vi "UHR-Fleezers Control (fpga) - 10.9.vi"() -> ()   [LabVIEW 2014]
doc: "UHR-Fleezers Instrument Control Code (fpga)"
uses:
  <vilib>/eio/EIONode/EIONode.xnode
  <vilib>/eio/EIOMethodNode/EIOMethodNode.xnode
  <vilib>/rvi/DataTransferAndStorage/Container/XNode/niFpgaContainer.xnode
  <vilib>/Platform/TimedLoop/XDataNode/XDataNode.xnode
  <vilib>/Platform/TimedLoop/XDataNode/nitl_modes.ctl
  <vilib>/Platform/TimedLoop/XDataNode/XDNodeRunTimeDep.lvlib
  <vilib>/Platform/TimedLoop/XDataNode/wakeup.ctl
  <vilib>/Platform/TimedLoop/XDataNode/timing_clust.ctl
  <vilib>/addons/control/pid/fpga.llb/XNode/niFpgaPID.xnode
  <vilib>/rvi/eio/common/nirviEmuTemplateMethod_errors.vi
  <vilib>/rvi/interface/RandomDataEmulation/nirviRandomDataFpgaReadWriteTemplate.vi
panel:
  in  "Connector0/AO6":i16
  in  "Tab Control":T1(tab)=enum."Force FB"
  in  "Trap Pos to FIFO":bool
  in  "AI1 Sets to FIFO":T2={"Set 1"=TRUE, "Set 2"=TRUE, "Set 3"=FALSE}
  in  "N of AI1 Int Acq Sets":i16=2 min=1 max=3 step=1
  out "AI Late Counter":u8
  in  "ai count":u16=400
  in  "+ phase":bool
  in  "Phase count adjustment":i16
  out "Relative phase":i16
  in  "AI to FIFO":bool
  out "BD1 Frequency Out 1":u64
  out "BD1 Frequency Out 2":u64
  out "Trap Pos FIFO Timeout":u16
  out "Trap AI FIFO Timeout":u16
  in  "Trap FIFO Set Timeout":i32
  in  "Tab Control 2":T3(tab)
  out "Wiggling 2":bool
  in  "Abort wiggle 2":bool
  in  "Wiggle amp 2":u64
  in  "Wiggle freq 2 (Hz)":fxp<+/-,16,16>
  in  "Wiggle trap 2":bool
  out "Wiggling 1":bool
  in  "Abort wiggle 1":bool
  in  "Wiggle trap 1":bool
  in  "Wiggle amp 1":u64
  in  "Wiggle freq 1 (Hz)":fxp<+/-,16,16>
  in  "Swap F1 and F2":bool
  in  "Freq or Amp switch first":bool=TRUE
  in  "Cont. Scan":bool
  in  "Abort scan":bool
  in  "Cycles per step":u64
  in  "Scan BD":bool
  in  "Number of scans":u16
  in  "Scan steps":u64
  in  "Scan freq.  increment":i64
  out "Scanning":bool
  in  "Start scan":bool
  in  "OSK Bd 1":bool
  in  "Reset Bd 1":bool
  in  "RD":bool
  in  "PMODE":bool
  in  "OSK Bd 2":bool
  in  "Reset Bd 2":bool
  in  "Direct RF Box \nCommunication":bool
  in  "Data BD 2":u8 format="%08b"
  in  "Data BD 1":u8 format="%08b"
  in  "Address":u8 format="%02x"
  in  "Update Data":bool
  in  "FPGA Controls\n RF Box":bool
  in  "Number Interlace Cycles":u8=2 min=1 max=3
  in  "Interlace Off Parameters":u8=1 min=1 max=3
  in  "Interlace ON/OFF":bool
  out "DIO Relative phase":i16
  in  "Phase count adjustment (DIO)":i16
  in  "+ phase (DIO)":bool
  out "DIO Late Counter":u8
  in  "DIO count 1 (ticks)":u16=400
  in  "DIO count 2 (ticks)":u16=400
  in  "DIO count 3 (ticks)":u16=400
  out "AI2 Y Sum Set 2":i16
  out "AI2 Y Sum Set 1":i16
  in  "FB Gains Set 1":T4={"proportional gain (Kc)"=10, "integral gain (Kc*Ts/Ti)"=5, "derivative gain (Kc*Td/Ts)"=0}
  in  "FB Setpoint Set 1":i16 min=0 step=1
  in  "FB Reset Set 1":bool
  in  "FB On/Off Set 1":bool
  in  "FB Reset Set 2":bool
  in  "FB On/Off Set 2":bool
  in  "FB Setpoint Set 2":i16 min=0 step=1
  in  "FB Gains Set 2":T4={"proportional gain (Kc)"=10, "integral gain (Kc*Ts/Ti)"=5, "derivative gain (Kc*Td/Ts)"=0}
  in  "FB output range 2":cluster{"output high":i16, "output low":i16}={"output high"=3000, "output low"=0}
  in  "FB output range 1":cluster{"output high":i16, "output low":i16}={"output high"=3000, "output low"=0}
  out "Scan I":u64
  in  "Amp switch delay":u16=5
  in  "Freq switch delay":u16
  in  "BD 2 Amplitude 1":u16
  in  "BD 1 Amplitude 1":u16
  in  "BD 2 Frequency 1":u64
  in  "BD 1 Frequency 1":u64
  in  "BD 2 Amplitude 2":u16
  in  "BD 1 Amplitude 2":u16
  in  "BD 2 Frequency 2":u64
  in  "BD 1 Frequency 2":u64
  in  "BD 2 Amplitude 3":u16
  in  "BD 1 Amplitude 3":u16
  in  "BD 2 Frequency 3":u64
  in  "BD 1 Frequency 3":u64
  in  "Negate Diff?":bool
  in  "Diff FB Measurement?":bool
  in  "FB Trig Integrate":u32=1
  out "TTrig?":bool
  in  "TTrig Negate Pos":bool=TRUE
  out "Trap Pos FB Int Signal":fxp<+/-,24,9> format="%.18g"
  out "Trap Pos FB Int-Norm Signal":fxp<+/-,16,1> format="%.16g"
  in  "FPGA TTrig Thresh":i64
  in  "FPGA Trap Trig":bool
  out "Trap Pos FB Action":i64
  in  "Trap Pos. FB Offset Factor":i64
  in  "Trap Pos. FB Mult Factor":i64=2
  in  "Trap Pos. FB Range":T5={"output high"=0.999969482421875, "output low"=-1.0}
  in  "Trap Pos. FB Gains":T6={"proportional gain (Kc)"=0.0, "integral gain (Kc*Ts/Ti)"=10.0, "derivative gain (Kc*Td/Ts)"=0.0} {"proportional gain (Kc)" format="%.11g"; "integral gain (Kc*Ts/Ti)" format="%.11g"; "derivative gain (Kc*Td/Ts)" format="%.11g"}
  in  "Trap Pos. FB Reset":bool
  in  "Trap Pos FB Monitor T1 or T2":bool
  in  "AI1 X Scale":u16
  in  "Trap Pos FB Int Count":u16=100
  in  "Trap Pos FB Negate Action":bool
  out "AI1 X Set 2":fxp<+/-,16,1>
  out "AI1 X Set 1":fxp<+/-,16,1>
  in  "Trap Pos. FB SP":fxp<+/-,16,1>
  in  "Force feedback":bool
  out "TTrig Sig":i64
  out "TTrig Fin Thresh":i64
  out "Numeric":i32
  out "AO2 2":i16
  out "AO1 2":i16
  in  "1D or 2D Scan?":bool
  in  "Abort scan (MCL)":bool
  in  "MCL Scan Axis":bool
  in  "Cont. Scan (MCL)":bool
  out "Scan I (MCL)":u64
  in  "Number of scans (MCL)":u16
  out "Scanning MCL":bool
  in  "Scan steps (MCL)":u64
  in  "Cycles per step (MCL)":u64
  in  "Scan freq.  increment (MCL)":i16
  in  "Start scan (MCL)":bool
  in  "AO2":i16
  in  "AO1":i16
  out "MCL Late Counter":u8
  in  "MCL count":u32=800
  out "MCL Relative Phase":i16
  in  "Phase count adjustment (MCL)":i16
  in  "+ phase (MCL)":bool
  in  "APD Gate Operating Mode":u8 max=2 step=1
  in  "Invert APD Gate":bool
  in  "APD Gate OFF Count":u16=100
  in  "APD Gate ON Count":u16=300
  out "APD 1 Gate Late Counter":u8
  out "APD 1 Gate Relative Phase":i16
  in  "Phase count adjustment (APD 1 Gate)":i16
  in  "+ phase (APD 1 Gate)":bool
  out "APD 2 Counts 0":u32
  out "APD 2 Counts 1":u32
  out "APD 1 Counts 0":u32
  out "APD 1 Counts 1":u32
  out "APD 1 out state":bool
  in  "APD 2 AO scale factor":i16=1
  in  "APD 1 AO scale factor":i16=1
  in  "APD to FIFO":bool
  in  "APD Acq Rate Count":u32=20000000
  out "APD Acq Late Counter":u8
  out "APD Acq Relative Phase":i16
  in  "Phase Count Adjustment (APD Acq)":i16
  in  "+ phase (APD Acq)":bool
  in  "Phase count adjustment (APD 2 Gate)":i16
  out "APD 2 Gate Late Counter":u8
  out "APD 2 Gate Relative Phase":i16
  in  "+ phase (APD 2 Gate)":bool
  out "APD 2 out state":bool
  out "APD 1 Int Gate":bool
  out "APD 2 Int Gate":bool
  in  "Green Filter Flipper":bool
  out "Green FB Signals":T7
  in  "Green FB Count":u16=1200
  out "Green Late Counter":u8
  out "Green FB Relative Phase":i16
  in  "Phase count adjustment (Green FB)":i16=10
  in  "+ phase (Green FB)":bool
  out "Green FB Sum":i16
  in  "Green int current ON count adj":u16=150
  in  "Current Out":u16=30000
  in  "Green FB On/Off":bool
  in  "Green FB Setpoint":i16=250 min=0 step=1
  in  "Green FB Gains":T4={"proportional gain (Kc)"=10, "integral gain (Kc*Ts/Ti)"=5, "derivative gain (Kc*Td/Ts)"=0}
  in  "Green FB Reset":bool
  in  "Operating Mode 2":u8=2 max=2 step=1
  in  "Invert GI 2":bool
  in  "Green interlace OFF count 2":u16=900
  in  "Green interlace ON count 2":u16=300
  out "GI Late Counter 2":u8
  out "GI Relative phase 2":i16
  in  "Phase count adjustment (GI) 2":i16=20
  in  "+ phase (GI) 2":bool
  in  "Green interlace OFF count":u16=100
  out "GI Relative phase":i16
  in  "Phase count adjustment (GI)":i16
  in  "+ phase (GI)":bool
  in  "Green interlace ON count":u16=300
  out "GI Late Counter":u8
  in  "Invert GI":bool
  in  "Operating Mode":u8 max=2 step=1
  in  "Red FB Reset":bool
  in  "Red FB Setpoint":i16
  in  "Red FB On/Off":bool
  in  "Invert RI 2":bool
  in  "Invert RI":bool
  in  "Phase count adjustment (RI)":i16
  in  "+ phase (RI)":bool
  in  "RI OFF count":u16
  in  "RI ON count":u16
  in  "RI Current Out":u16
  in  "RI operating mode 2":u8
  in  "Red operating mode":u8
  out "RI late counter":u8
  out "RI relative phase":i16
  out "Red FB Sum":i16
  in  "Red FB Gains":T4={"proportional gain (Kc)"=1, "integral gain (Kc*Ts/Ti)"=0, "derivative gain (Kc*Td/Ts)"=0}
  in  "Chassis2/Mod4/AO1":u16
  # "Only one of these can be on\nat a time:"
  # "Raster Scan AOD"
  # "1 (X)"
  # "2 (Y)"
  # "IR Intensity Feedback (RF BD 1)"
  # "FB Triggering Excitation Laser"
  # "AO1 (Y)"
  # "2D"
  # "1D"
  # "AO2 (X)"
  # "APD AO for aligning"
  # "Detection Loop"
  # "Green fluorescent laser digital gate interlacing loop"
  # "0 Forced ON\n1 Forced OFF\n2 Interlacing"
  # "Red fluorescent laser digital gate interlacing loop"
  # "0 Forced ON\n1 Forced OFF\n2 Interlacing"
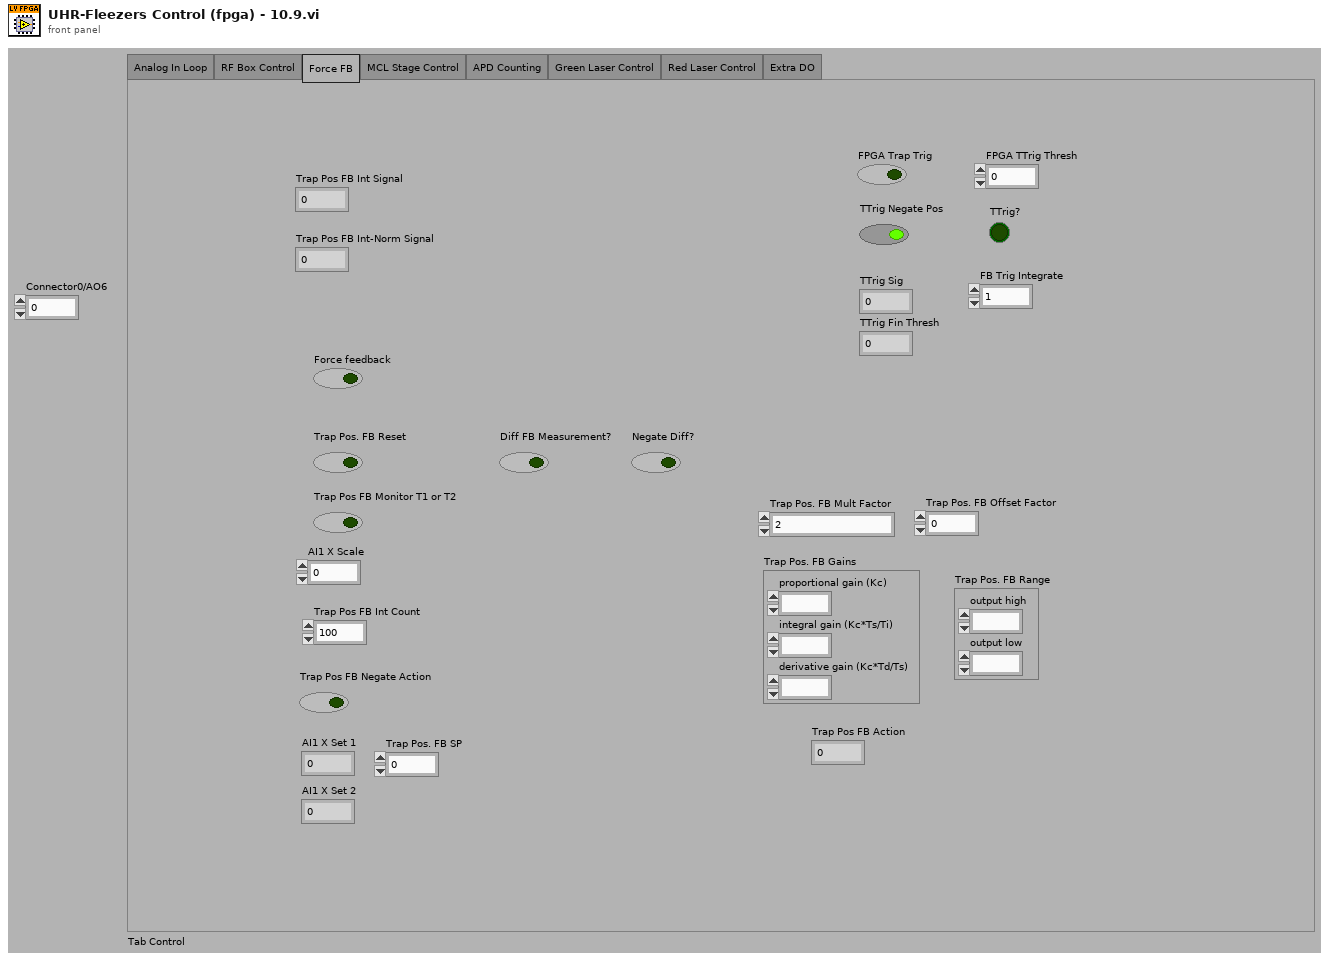
[diagram p1: front panel]
types:
  T1 = enum32{"Analog In Loop", "RF Box Control", "Force FB", "MCL Stage Control", "APD Counting", "Green Laser Control", "Red Laser Control", "Extra DO"}
  T2 = cluster{"Set 1":bool, "Set 2":bool, "Set 3":bool}
  T3 = enum32{"Controls", "Interlacing Frequency and Amplitude Values"}
  T4 = cluster{"proportional gain (Kc)":i16, "integral gain (Kc*Ts/Ti)":i16, "derivative gain (Kc*Td/Ts)":i16}
  T5 = cluster{"output high":fxp<+/-,16,1>, "output low":fxp<+/-,16,1>}
  T6 = cluster{"proportional gain (Kc)":fxp<+/-,16,8>, "integral gain (Kc*Ts/Ti)":fxp<+/-,16,8>, "derivative gain (Kc*Td/Ts)":fxp<+/-,16,8>}
  T7 = cluster{"Green FB Ch 0":i16, "Green FB Ch 1":i16, "Green FB Ch 2":i16}
  T8 = typedef "XDNodeRunTimeDep.lvlib/timing_clust.ctl" = cluster{"Expected End [f-1]":u64, "Actual End [f-1]":u64, "Finished Late? [f-1]":bool, "Expected End [i-1]":u64, "Actual End [i-1]":u64, "Finished Late? [i-1]":bool, "Expected Start [i]":u64, "Actual Start [i]":u64, "Expected Start [f]":u64, "Actual Start [f]":u64, "Source Name":string, "Structure Name":string, "Period":i64, "Deadline":i64, "Offset":i64, "Start":i64, "Priority":i32, "Timeout":i32, "Mode":T9, "Wakeup Reason":T10, "Error":errorcluster, "Source Type":string, "Secondary Source Type":string, "Global End Time":u64, "Global Start Time":u64, "Frame Duration":u64, "Iteration Duration":u64, "Assigned CPU":i32, "I/O Scan Engine Mode":u32}
  T9 = typedef "XDNodeRunTimeDep.lvlib/nitl_modes.ctl" = enum32{"No Change", "Process missed periods, maintain original phase", "Discard missed periods, maintain original phase", "Process missed periods, ignore original phase", "Discard missed periods, ignore original phase"}
  T10 = typedef "XDNodeRunTimeDep.lvlib/wakeup.ctl" = enum32{"Normal", "Aborted", "Asynchronous wakeup", "Timing source error", "Timed loop error", "Timeout"}
  T11 = cluster{"Chassis2/Mod1/AI0":void, "Chassis2/Mod1/AI1":void, "Chassis2/Mod1/AI2":void}
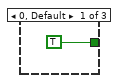
[diagram p2: hidden frame]
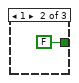
[diagram p3: hidden frame]
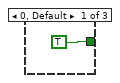
[diagram p4: hidden frame]
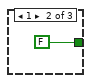
[diagram p5: hidden frame]
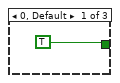
[diagram p7: hidden frame]
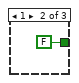
[diagram p8: hidden frame]
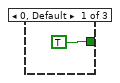
[diagram p10: hidden frame]
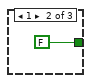
[diagram p11: hidden frame]
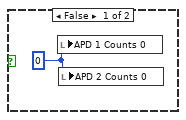
[diagram p12: hidden frame]
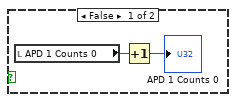
[diagram p15: hidden frame]
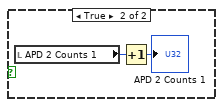
[diagram p17: hidden frame]
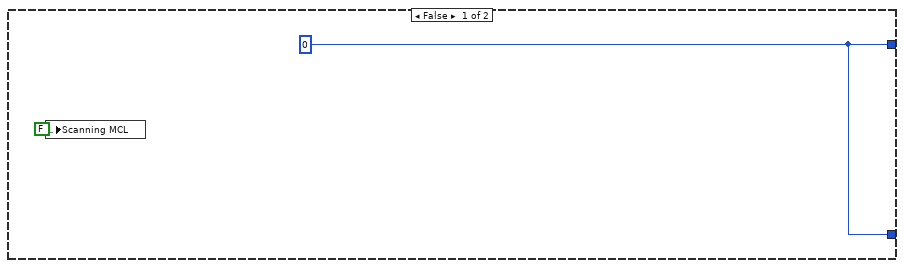
[diagram p18: hidden frame]
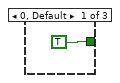
[diagram p19: hidden frame]
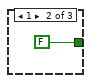
[diagram p20: hidden frame]
diagram:
  w1 = u16 0
  w4 = FALSE
  w2 = FALSE
  # "633 nm red excitation laser interlacing (DO to IA 633 nm AOM ME amp)."
  # "The APD Int Gate is here so the FPGA will do the integration only when the APD gate is \"ON\" (though we will leave the APD continuously ON now). This was added because the actual APD gating (via the hardware) was giving false signals. -KW"
  # "timing array current index"
  # "timing array"
  # "timing counter (phase adjusted here)"
  # "late counter"
  n1 = flat-sequence "FPGA initialization to do before running any of the loops" {
    tunnel: [u16 0 ("DIO count 3 (ticks)")] -> w3
    tunnel: [w10] -> _
    frame #0 {
      # "Start up expansion chassis early\nto avoid delays later"
      # "This pin controls udclk on the RF boards.\nWhen initially configuring the boards, this pin needs to be\nconfigured as a high impedance input.  Later it will be switched\nto an output."
      # "Initial setting of DIO data and \naddress to low (before reset).  \nThis needs to happen before the other\ncontrol method loops execute."
      n2 = xnode "FPGA I/O Node"("Chassis2/Mod4/AO0"=u16 0) -> ("Chassis2/Mod1/AI0"=w10)  [unwired: 2 in, 2 out]
      n3 = xnode "FPGA I/O Method Node"("Enable"=FALSE) -> ()  [unwired: 1 in, 1 out]
      n4 = xnode "FPGA I/O Node"("Connector1/DIO0"=FALSE, "Connector1/DIO1"=FALSE, "Connector1/DIO2"=FALSE, "Connector1/DIO3"=FALSE, "Connector1/DIO4"=FALSE, "Connector1/DIO5"=FALSE, "Connector1/DIO6"=FALSE, "Connector1/DIO7"=FALSE, "Connector1/DIO8"=FALSE, "Connector1/DIO9"=FALSE, "Connector1/DIO10"=FALSE, "Connector1/DIO11"=FALSE, "Connector1/DIO12"=FALSE, "Connector1/DIO13"=FALSE, "Connector1/DIO15"=FALSE, "Connector1/DIO20"=FALSE, "Connector1/DIO21"=FALSE, "Connector1/DIO22"=FALSE, "Connector1/DIO23"=FALSE, "Connector1/DIO24"=FALSE, "Connector1/DIO25"=FALSE, "Connector1/DIO26"=FALSE, "Connector1/DIO27"=FALSE, "Connector1/DIO14"=FALSE) -> ()  [unwired: 24 in, 24 out]
    }
  }
  n5 = local read "AO1"() -> (w8:i16)
  n6 = local read "AO2"() -> (w7:i16)
  n7 = node-c288() -> (w6:T8)  [unwired: 1 in]
  n8 = while "APD 1 Counter" {
    tunnel: w3 -> [_]
    stop <- FALSE stop-if-true
    n9 = flat-sequence {
      frame #0 {
        n10 = xnode "FPGA I/O Method Node"("FPGA I/O In"=refnum<k21> "Connector0/DIO0" ("APD 1 DO"), "Timeout"=-1) -> ()  [unwired: 2 out]
      }
      frame #1 {
        n11 = local read "APD 1 Int Gate"() -> (w41:bool)
        n12 = case shown="True" w41 {
          frame False {
          }
          frame True {
            n13 = local read "APD 1 out state"() -> (w42:bool)
            n14 = case shown="True" w42 {
              frame False {
                n15 = local read "APD 1 Counts 0"() -> (w44:u32)
                n16 = Increment(x=w44) -> (x+1=→"APD 1 Counts 0":u32)
              }
              frame True {
                n17 = local read "APD 1 Counts 1"() -> (w46:u32)
                n18 = Increment(x=w46) -> (x+1=→"APD 1 Counts 1":u32)
              }
            }
          }
        }
      }
    }
  }
  n19 = while "APD 2 Counter" {
    tunnel: w3 -> [_]
    stop <- FALSE stop-if-true
    n20 = flat-sequence {
      frame #0 {
        n21 = xnode "FPGA I/O Method Node"("FPGA I/O In"=refnum<k21> "Connector0/DIO1" ("APD 2 DO"), "Timeout"=-1) -> ()  [unwired: 2 out]
      }
      frame #1 {
        n22 = local read "APD 2 Int Gate"() -> (w50:bool)
        n23 = case shown="True" w50 {
          frame False {
          }
          frame True {
            n24 = local read "APD 2 out state"() -> (w51:bool)
            n25 = case shown="False" w51 {
              frame False {
                n26 = local read "APD 2 Counts 0"() -> (w53:u32)
                n27 = Increment(x=w53) -> (x+1=→"APD 2 Counts 0":u32)
              }
              frame True {
                n28 = local read "APD 2 Counts 1"() -> (w55:u32)
                n29 = Increment(x=w55) -> (x+1=→"APD 2 Counts 1":u32)
              }
            }
          }
        }
      }
    }
  }
  n30 = while "APD 2 Gating" {
    shift-right: [w59] -> _
    shift-left: w3 -> [w64]
    shift-right: [w58] -> _
    shift-left: w4 -> [w56]
    stop <- FALSE stop-if-true
    n31 = flat-sequence {
      tunnel: w64 -> [w67]
      tunnel: [w68] -> w62
      tunnel: [w67] -> w60
      tunnel: [w66] -> w57
      tunnel: w56 -> [w66]
      tunnel: [w71] -> w63
      tunnel: w62 -> [w71]
      tunnel: [w70] -> w61
      tunnel: w60 -> [w70]
      tunnel: w57 -> [w69]
      tunnel: [w89] -> w59
      tunnel: w63 -> [w100]
      tunnel: w61 -> [w98]
      tunnel: [w93] -> w58
      frame #0 {
        n32 = call "Loop Timer8"("Count(Ticks)"=w67) -> ("Tick Count(Ticks)"=w68:u16)
      }
      frame #1 {
        # "(need 4 channels/APD)"
        n33 = xnode "FPGA I/O Node"("Connector0/DIO8"=w69, "Connector0/DIO9"=w69, "Connector0/DIO10"=w69, "Connector0/DIO11"=w69) -> ()  [unwired: 4 in, 4 out]
        "APD 2 Int Gate" <- w69
      }
      frame #2 {
        n34 = local read "APD Gate ON Count"() -> (w82:u16)
        n35 = local read "APD Gate OFF Count"() -> (w81:u16)
        n36 = feedback #1(TRUE) -> (w95:bool)
        n37 = feedback-in #2(w100) -> ()
        n38 = feedback #2(w100) -> (w83:u16)
        n39 = Not(x=w95) -> (.not. x?=w92:bool)
        n40 = feedback-in #1(w92) -> ()
        n41 = Subtract(x=w100, y=w83) -> (x-y=w99:u16)
        n42 = Select(t=w82, s=w92, f=w81) -> (s? t:f=w97:u16)
        n43 = Subtract(x=w99, y=w98) -> (x-y=w74:u16)
        n44 = Subtract(x=w97, y=w74) -> (x-y=w88:u16)
        n45 = Number To Boolean Array(number=w74) -> (Boolean array=w73:bool[])
        n46 = Or Array Elements(Boolean array=w73) -> (logical OR=w72:bool)
        n47 = Boolean To (0,1)(Boolean="+ phase (APD 2 Gate)") -> (0, 1=w86:i16)
        n48 = Multiply(x=w86, y="Phase count adjustment (APD 2 Gate)") -> (x*y=w84:i16)
        n49 = Boolean To (0,1)(Boolean=w72) -> (0, 1=w79:i16)
        n50 = Add(x=w88, y=w84) -> (x+y=w89:u16)
        n51 = To Unsigned Byte Integer(number=w79) -> (unsigned 8bit integer=w76:u8)
        n52 = feedback #3(i16 0) -> (w91:i16)
        n53 = Subtract(x=w91, y=w84) -> (x-y=w90:i16)
        "APD 2 Gate Relative Phase" <- w90
        n54 = feedback-in #3(w90) -> ()
        n55 = feedback #4(u8 0) -> (w77:u8)
        n56 = Add(x=w76, y=w77) -> (x+y=w75:u8)
        "APD 2 Gate Late Counter" <- w75
        n57 = feedback-in #4(w75) -> ()
        n58 = local read "APD Gate Operating Mode"() -> (w80:u8)
        n59 = case shown="2" w80 {
          tunnel: [TRUE FALSE w106] -> w93
          tunnel: w95 -> [_ _ w104]
          frame 0, Default {
          }
          frame 1 {
          }
          frame 2 {
            n60 = local read "Invert APD Gate"() -> (w103:bool)
            n61 = Not(x=w104) -> (.not. x?=w105:bool)
            n62 = Select(t=w105, s=w103, f=w104) -> (s? t:f=w106:bool)
          }
        }
      }
    }
  }
  n63 = while "APD 1 Gating" {
    shift-right: [w110] -> _
    shift-left: w3 -> [w115]
    shift-right: [w109] -> _
    shift-left: w4 -> [w107]
    stop <- FALSE stop-if-true
    n64 = flat-sequence {
      tunnel: w115 -> [w118]
      tunnel: [w119] -> w113
      tunnel: [w118] -> w111
      tunnel: [w117] -> w108
      tunnel: w107 -> [w117]
      tunnel: [w122] -> w114
      tunnel: w113 -> [w122]
      tunnel: [w121] -> w112
      tunnel: w111 -> [w121]
      tunnel: w108 -> [w120]
      tunnel: [w136] -> w110
      tunnel: w114 -> [w151]
      tunnel: w112 -> [w148]
      tunnel: [w140] -> w109
      frame #0 {
        n65 = call "Loop Timer7"("Count(Ticks)"=w118) -> ("Tick Count(Ticks)"=w119:u16)
      }
      frame #1 {
        # "(need 4 channels/APD)"
        n66 = xnode "FPGA I/O Node"("Connector0/DIO4"=w120, "Connector0/DIO5"=w120, "Connector0/DIO6"=w120, "Connector0/DIO7"=w120) -> ()  [unwired: 4 in, 4 out]
        "APD 1 Int Gate" <- w120
      }
      frame #2 {
        n67 = feedback #5(TRUE) -> (w143:bool)
        n68 = feedback-in #6(w151) -> ()
        n69 = feedback #6(w151) -> (w150:u16)
        n70 = Not(x=w143) -> (.not. x?=w139:bool)
        n71 = feedback-in #5(w139) -> ()
        n72 = Subtract(x=w151, y=w150) -> (x-y=w149:u16)
        n73 = Select(t="APD Gate ON Count", s=w139, f="APD Gate OFF Count") -> (s? t:f=w145:u16)
        n74 = Subtract(x=w149, y=w148) -> (x-y=w124:u16)
        n75 = Subtract(x=w145, y=w124) -> (x-y=w135:u16)
        n76 = Number To Boolean Array(number=w124) -> (Boolean array=w125:bool[])
        n77 = Or Array Elements(Boolean array=w125) -> (logical OR=w123:bool)
        n78 = Boolean To (0,1)(Boolean="+ phase (APD 1 Gate)") -> (0, 1=w133:i16)
        n79 = Boolean To (0,1)(Boolean=w123) -> (0, 1=w130:i16)
        n80 = Multiply(x=w133, y="Phase count adjustment (APD 1 Gate)") -> (x*y=w131:i16)
        n81 = To Unsigned Byte Integer(number=w130) -> (unsigned 8bit integer=w127:u8)
        n82 = Add(x=w135, y=w131) -> (x+y=w136:u16)
        n83 = feedback #7(i16 0) -> (w138:i16)
        n84 = Subtract(x=w138, y=w131) -> (x-y=w137:i16)
        "APD 1 Gate Relative Phase" <- w137
        n85 = feedback-in #7(w137) -> ()
        n86 = feedback #8(u8 0) -> (w128:u8)
        n87 = Add(x=w127, y=w128) -> (x+y=w126:u8)
        "APD 1 Gate Late Counter" <- w126
        n88 = feedback-in #8(w126) -> ()
        n89 = case shown="2" "APD Gate Operating Mode" {
          tunnel: [TRUE FALSE w157] -> w140
          tunnel: w143 -> [_ _ w154]
          frame 0, Default {
          }
          frame 1 {
          }
          frame 2 {
            n90 = Not(x=w154) -> (.not. x?=w156:bool)
            n91 = Select(t=w156, s="Invert APD Gate", f=w154) -> (s? t:f=w157:bool)
          }
        }
      }
    }
  }
  n92 = timed-loop "RF box board DIO control: control bits" {
    timing: w6 -> [_]
    timing-out: [_] -> w5
    tunnel: [w158] -> _
    tunnel: w3 -> [w158]
    stop <- FALSE stop-if-true
    n93 = xnode "FPGA I/O Node"("Connector1/DIO16"="RD", "Connector1/DIO17"="PMODE", "Connector1/DIO18"="OSK Bd 1", "Connector1/DIO19"="Reset Bd 1", "Connector1/DIO28"="OSK Bd 2", "Connector1/DIO29"="Reset Bd 2") -> ()  [unwired: 6 in, 6 out]
  }
  n94 = while "532 nm green excitation laser interlacing (DO to IA 532 nm AOM ME amp)." {
    shift-right: [w171] -> _
    shift-left: w3 -> [w176]
    shift-right: [w170] -> _
    shift-left: w2 -> [w168]
    stop <- FALSE stop-if-true
    n95 = flat-sequence {
      tunnel: w176 -> [w179]
      tunnel: [w180] -> w174
      tunnel: [w179] -> w172
      tunnel: [w178] -> w169
      tunnel: w168 -> [w178]
      tunnel: [w183] -> w175
      tunnel: w174 -> [w183]
      tunnel: [w182] -> w173
      tunnel: w172 -> [w182]
      tunnel: w169 -> [w181]
      tunnel: [w192] -> w171
      tunnel: w175 -> [w212]
      tunnel: w173 -> [w209]
      tunnel: [w201] -> w170
      frame #0 {
        n96 = call "Loop Timer4"("Count(Ticks)"=w179) -> ("Tick Count(Ticks)"=w180:u16)
      }
      frame #1 {
        n97 = xnode "FPGA I/O Node"("Connector1/DIO37"=w181, "Connector1/DIO38"=w181, "Connector1/DIO39"=w181) -> ()  [unwired: 3 in, 3 out]
      }
      frame #2 {
        n98 = feedback-in #9(w212) -> ()
        n99 = feedback #9(w212) -> (w211:u16)
        n100 = Subtract(x=w212, y=w211) -> (x-y=w210:u16)
        n101 = Subtract(x=w210, y=w209) -> (x-y=w185:u16)
        n102 = Number To Boolean Array(number=w185) -> (Boolean array=w186:bool[])
        n103 = Or Array Elements(Boolean array=w186) -> (logical OR=w184:bool)
        n104 = Boolean To (0,1)(Boolean="+ phase (GI)") -> (0, 1=w197:i16)
        n105 = Multiply(x=w197, y="Phase count adjustment (GI)") -> (x*y=w194:i16)
        n106 = Boolean To (0,1)(Boolean=w184) -> (0, 1=w191:i16)
        n107 = To Unsigned Byte Integer(number=w191) -> (unsigned 8bit integer=w188:u8)
        n108 = feedback #10(i16 0) -> (w195:i16)
        n109 = feedback #11(u8 0) -> (w189:u8)
        n110 = Add(x=w188, y=w189) -> (x+y=w187:u8)
        "GI Late Counter" <- w187
        n111 = feedback-in #11(w187) -> ()
        n112 = Subtract(x=w195, y=w194) -> (x-y=w193:i16)
        "GI Relative phase" <- w193
        n113 = feedback-in #10(w193) -> ()
        n114 = feedback #12(TRUE) -> (w204:bool)
        n115 = case shown="2" "Operating Mode" {
          tunnel: [TRUE FALSE w218] -> w201
          tunnel: w204 -> [_ _ w215]
          frame 0, Default {
          }
          frame 1 {
          }
          frame 2 {
            n116 = Not(x=w215) -> (.not. x?=w217:bool)
            n117 = Select(t=w217, s="Invert GI", f=w215) -> (s? t:f=w218:bool)
          }
        }
        n118 = Not(x=w204) -> (.not. x?=w200:bool)
        n119 = Select(t="Green interlace ON count", s=w200, f="Green interlace OFF count") -> (s? t:f=w206:u16)
        n120 = Subtract(x=w206, y=w185) -> (x-y=w198:u16)
        n121 = Add(x=w198, y=w194) -> (x+y=w192:u16)
        n122 = feedback-in #12(w200) -> ()
      }
    }
  }
  n123 = while "Green and red excitation laser interlacing (Current AO to IA 532 nm AOM ME amp)." {
    shift-right: [w227] -> _
    shift-left: w3 -> [w230]
    shift-right: [w224] -> _
    shift-left: w1 -> [w222]
    shift-right: [w219] -> _
    shift-left: w1 -> [w221]
    stop <- FALSE stop-if-true
    n124 = flat-sequence {
      tunnel: w230 -> [w234]
      tunnel: [w235] -> w229
      tunnel: [w234] -> w228
      tunnel: [w233] -> w223
      tunnel: w222 -> [w233]
      tunnel: w221 -> [w232]
      tunnel: [w232] -> w220
      tunnel: [w239] -> w226
      tunnel: w229 -> [w239]
      tunnel: [w238] -> w225
      tunnel: w228 -> [w238]
      tunnel: w223 -> [w237]
      tunnel: w220 -> [w236]
      tunnel: [w259] -> w227
      tunnel: [w276] -> w224
      tunnel: w226 -> [w245]
      tunnel: w225 -> [w285]
      tunnel: [w247] -> w219
      frame #0 {
        n125 = call "Loop Timer10"("Count(Ticks)"=w234) -> ("Tick Count(Ticks)"=w235:u16)
      }
      frame #1 {
        n126 = xnode "FPGA I/O Node"("Chassis2/Mod4/AO0"=w237, "Chassis2/Mod4/AO1"=w236) -> ()  [unwired: 2 in, 2 out]
      }
      frame #2 {
        # "Design note (Comstock lab):\n\nThese two laser controls are in the same loop\nbecause the expansion current AI cannot separately\ntime the outputs fast enough for us.  Apparently\nit is because of communication time between the\nexpansion card and the fpga.\n\nSo the two analog control signals have the same timing\nand profile, but independent amplitudes to independently\ncontrol the intensity and feedback for each laser."
        n127 = feedback #13(TRUE) -> (w246:bool)
        n128 = Subtract(x="Green interlace OFF count 2", y="Green int current ON count adj") -> (x-y=w268:u16)
        n129 = Not(x=w246) -> (.not. x?=w278:bool)
        n130 = feedback-in #13(w278) -> ()
        n131 = feedback-in #14(w245) -> ()
        n132 = feedback #14(w245) -> (w287:u16)
        n133 = Add(x="Green int current ON count adj", y="Green interlace ON count 2") -> (x+y=w269:u16)
        n134 = Subtract(x=w245, y=w287) -> (x-y=w286:u16)
        n135 = Select(t=w269, s=w278, f=w268) -> (s? t:f=w282:u16)
        n136 = Subtract(x=w286, y=w285) -> (x-y=w252:u16)
        n137 = case shown="2" "RI operating mode 2" {
          tunnel: [TRUE FALSE w301] -> w242
          tunnel: w246 -> [_ _ w303]
          frame 0, Default {
          }
          frame 1 {
          }
          frame 2 {
            n138 = Not(x=w303) -> (.not. x?=w302:bool)
            n139 = Select(t=w302, s="Invert RI 2", f=w303) -> (s? t:f=w301:bool)
          }
        }
        n140 = case shown="2" "Operating Mode 2" {
          tunnel: [TRUE FALSE w321] -> w270
          tunnel: w246 -> [_ _ w318]
          frame 0, Default {
          }
          frame 1 {
          }
          frame 2 {
            n141 = Not(x=w318) -> (.not. x?=w320:bool)
            n142 = Select(t=w320, s="Invert GI 2", f=w318) -> (s? t:f=w321:bool)
          }
        }
        n143 = Subtract(x=w282, y=w252) -> (x-y=w263:u16)
        n144 = Number To Boolean Array(number=w252) -> (Boolean array=w253:bool[])
        n145 = Boolean To (0,1)(Boolean="+ phase (GI) 2") -> (0, 1=w265:i16)
        n146 = Or Array Elements(Boolean array=w253) -> (logical OR=w251:bool)
        n147 = Boolean To (0,1)(Boolean=w251) -> (0, 1=w258:i16)
        n148 = Multiply(x=w265, y="Phase count adjustment (GI) 2") -> (x*y=w261:i16)
        n149 = To Unsigned Byte Integer(number=w258) -> (unsigned 8bit integer=w254:u8)
        n150 = Add(x=w263, y=w261) -> (x+y=w259:u16)
        n151 = feedback #15(u8 0) -> (w256:u8)
        n152 = Add(x=w254, y=w256) -> (x+y=w255:u8)
        "GI Late Counter 2" <- w255
        n153 = feedback-in #15(w255) -> ()
        n154 = feedback #16(i16 0) -> (w262:i16)
        n155 = Subtract(x=w262, y=w261) -> (x-y=w260:i16)
        "GI Relative phase 2" <- w260
        n156 = feedback-in #16(w260) -> ()
        n157 = And(x=w270, y="Green FB On/Off") -> (x .and. y?=w271:bool)
        n158 = case shown="True" w271 {
          tunnel: "Current Out" -> [w305 _]
          tunnel: [w305 w310] -> w275
          frame False {
          }
          frame True {
            n159 = local read "Green FB Sum"() -> (w306:i16)
            n160 = call "Slower PID.vi"("process variable"=w306, "reset?"="Green FB Reset", "setpoint"="Green FB Setpoint", "PID gains (x 2^8)"="Green FB Gains", "output range"=cluster{"output high":i16, "output low":i16} {"output high"=32767, "output low"=-32768} ("Green FB output range")) -> ("output"=w314:i16)  [unwired: 10 out]
            n161 = To Long Integer(number=w314) -> (32bit integer=w307:i32)
            n162 = Add(x=w307, y=32768) -> (x+y=w309:i32)
            n163 = To Unsigned Word Integer(number=w309) -> (unsigned 16bit integer=w310:u16)
          }
        }
        n164 = And(x=w242, y="Red FB On/Off") -> (x .and. y?=w240:bool)
        n165 = case shown="True" w240 {
          tunnel: "RI Current Out" -> [w288 _]
          tunnel: [w288 w289] -> w243
          frame False {
          }
          frame True {
            n166 = local read "Red FB Sum"() -> (w296:i16)
            n167 = call "Slower PID.vi"("process variable"=w296, "reset?"="Red FB Reset", "setpoint"="Red FB Setpoint", "PID gains (x 2^8)"="Red FB Gains", "output range"=cluster{"output high":i16, "output low":i16} {"output high"=32767, "output low"=-32768} ("Green FB output range")) -> ("output"=w293:i16)  [unwired: 10 out]
            n168 = To Long Integer(number=w293) -> (32bit integer=w292:i32)
            n169 = Add(x=w292, y=32768) -> (x+y=w290:i32)
            n170 = To Unsigned Word Integer(number=w290) -> (unsigned 16bit integer=w289:u16)
          }
        }
        n171 = Boolean To (0,1)(Boolean=w270) -> (0, 1=w277:i16)
        n172 = Boolean To (0,1)(Boolean=w242) -> (0, 1=w249:i16)
        n173 = To Unsigned Word Integer(number=w277) -> (unsigned 16bit integer=w274:u16)
        n174 = To Unsigned Word Integer(number=w249) -> (unsigned 16bit integer=w248:u16)
        n175 = Multiply(x=w274, y=w275) -> (x*y=w276:u16)
        n176 = Multiply(x=w248, y=w243) -> (x*y=w247:u16)
      }
    }
  }
  n177 = while "Green excitation laser feedback measurement" {
    shift-right: [w322] -> _
    shift-left: w3 -> [w327]
    stop <- FALSE stop-if-true
    n178 = flat-sequence {
      tunnel: w327 -> [w329]
      tunnel: [w330] -> w325
      tunnel: [w329] -> w323
      tunnel: [w337] -> w326
      tunnel: w325 -> [w337]
      tunnel: [w336] -> w324
      tunnel: w323 -> [w336]
      tunnel: [w349] -> w322
      tunnel: w326 -> [w360]
      tunnel: w324 -> [w357]
      frame #0 {
        n179 = call "Loop Timer9"("Count(Ticks)"=w329) -> ("Tick Count(Ticks)"=w330:u16)
      }
      frame #1 {
        # "Design note (Comstock lab, MSU):\n\nAll lasers need to be measured at the same \ntime because the AI expansion module\ncannot independently time the measurements\nwithin our requirements: their is dead time.\n\nThis probably wouldn't be an issue with the built\nin AI on the fpga board itself."
        n180 = xnode "FPGA I/O Node"("Connector1/DIO35"=TRUE) -> ("Chassis2/Mod1/AI0"=w335, "Chassis2/Mod1/AI1"=w334, "Chassis2/Mod1/AI2"=w331)  [unwired: 4 in, 4 out]
        "Green FB Sum" <- w331
        "Red FB Sum" <- w335
        n181 = Bundle("Chassis2/Mod1/AI0"=w335, "Chassis2/Mod1/AI1"=w334, "Chassis2/Mod1/AI2"=w331) -> (→"Green FB Signals":T11)  [unwired: 1 out]
      }
      frame #2 {
        n182 = feedback-in #17(w360) -> ()
        n183 = feedback #17(w360) -> (w359:u16)
        n184 = Subtract(x=w360, y=w359) -> (x-y=w358:u16)
        n185 = xnode "FPGA I/O Node"("Connector1/DIO35"=FALSE) -> ()  [unwired: 1 in, 1 out]
        n186 = Subtract(x=w358, y=w357) -> (x-y=w339:u16)
        n187 = Subtract(x="Green FB Count", y=w339) -> (x-y=w353:u16)
        n188 = Number To Boolean Array(number=w339) -> (Boolean array=w340:bool[])
        n189 = Or Array Elements(Boolean array=w340) -> (logical OR=w338:bool)
        n190 = Boolean To (0,1)(Boolean="+ phase (Green FB)") -> (0, 1=w351:i16)
        n191 = Boolean To (0,1)(Boolean=w338) -> (0, 1=w345:i16)
        n192 = Multiply(x=w351, y="Phase count adjustment (Green FB)") -> (x*y=w346:i16)
        n193 = Add(x=w353, y=w346) -> (x+y=w349:u16)
        n194 = To Unsigned Byte Integer(number=w345) -> (unsigned 8bit integer=w342:u8)
        n195 = feedback #18(i16 0) -> (w348:i16)
        n196 = Subtract(x=w348, y=w346) -> (x-y=w347:i16)
        "Green FB Relative Phase" <- w347
        n197 = feedback-in #18(w347) -> ()
        n198 = feedback #19(u8 0) -> (w343:u8)
        n199 = Add(x=w342, y=w343) -> (x+y=w341:u8)
        "Green Late Counter" <- w341
        n200 = feedback-in #19(w341) -> ()
      }
    }
  }
  n201 = while "Control Additional IO (Green laser flip mount)" {
    stop <- FALSE stop-if-true
    n202 = xnode "FPGA I/O Node"("Connector0/DIO3"="Green Filter Flipper", "Chassis2/Mod4/AO1"="Chassis2/Mod4/AO1", "Connector0/AO6"="Connector0/AO6") -> ()  [unwired: 3 in, 3 out]
    n203 = call "Loop Timer2"("Count(Ticks)"=u32 40000 ("Extra DO Counts")) -> ()  [unwired: 1 out]
  }
  n204 = while "DAQ AI set 1" {
    shift-right: [w366] -> _
    shift-left: w3 -> [w371]
    stop <- FALSE stop-if-true
    n205 = flat-sequence {
      tunnel: w371 -> [w381]
      tunnel: [w382] -> w369
      tunnel: [w381] -> w368
      tunnel: [w392] -> w379
      tunnel: [w391] -> w378
      tunnel: [w390] -> w377
      tunnel: [w389] -> w376
      tunnel: [w388] -> w375
      tunnel: [w387] -> w374
      tunnel: [w386] -> w373
      tunnel: [w385] -> w372
      tunnel: [w384] -> w370
      tunnel: w369 -> [w384]
      tunnel: w368 -> [w383]
      tunnel: [w383] -> w367
      tunnel: [w421] -> w366
      tunnel: w379 -> [w449]
      tunnel: w378 -> [w413]
      tunnel: w377 -> [w414]
      tunnel: w376 -> [w448]
      tunnel: w375 -> [w437]
      tunnel: w374 -> [w436]
      tunnel: w373 -> [w435]
      tunnel: w372 -> [w434]
      tunnel: w370 -> [w431]
      tunnel: w367 -> [w428]
      frame #0 {
        n206 = call "Loop Timer3"("Count(Ticks)"=w381) -> ("Tick Count(Ticks)"=w382:u16)
      }
      frame #1 {
        n207 = xnode "FPGA I/O Node"("Connector1/DIO31"=TRUE ("Connector1/DIO33")) -> ("Connector0/AI0"=w392, "Connector0/AI1"=w391, "Connector0/AI2"=w390, "Connector0/AI3"=w389, "Connector0/AI4"=w388, "Connector0/AI5"=w387, "Connector0/AI6"=w386, "Connector0/AI7"=w385)  [unwired: 9 in, 9 out]
      }
      frame #2 {
        w417 = FALSE ("AI to FIFO")
        # "Adjust phase after data acquired if button pressed"
        n208 = feedback #20(i16 1) -> (w441:i16)
        n209 = Increment(x=w441) -> (x+1=w447:i16)
        n210 = Scale By Power Of 2(n="AI1 X Scale", x=w413) -> (x*2^n=w411:dbl)
        n211 = Greater?(x=w447, y="N of AI1 Int Acq Sets") -> (0:w444:bool)
        n212 = Select(t=i16 1, s=w444, f=w447) -> (s? t:f=w446:i16)
        n213 = feedback-in #20(w446) -> ()
        n214 = Divide(x=w411, y=w414) -> (x/y=w410:fxp<+/-,16,1>)
        n215 = feedback #21(w417) -> (w415:bool)
        n216 = feedback #22(w417) -> (w433:bool)
        n217 = case shown="1, Default" w441 {
          tunnel: w414 -> [w471 w479 _]
          tunnel: "AI1 Sets to FIFO" -> [w475 w483 w489]
          tunnel: [w474 w482 w488] -> w438
          tunnel: ["AI to FIFO" w481 w487] -> w432
          tunnel: w433 -> [_ w481 w487]
          tunnel: ["Trap Pos to FIFO" w480 w486] -> w416
          tunnel: w415 -> [_ w480 w486]
          tunnel: w410 -> [w470 w478 _]
          tunnel: [w469 w476 FALSE] -> w397
          tunnel: [w468 w477 u64 0 ("BD1 Frequency Out 2")] -> w396
          frame 1, Default {
            n218 = Unbundle By Name(w475) -> ("Set 1"=w474:bool)
            n219 = local read "BD1 Frequency Out 1"() -> (w468:u64)
            n220 = Compound Arithmetic op=AND("Trap Pos to FIFO", w474, "AI to FIFO") -> (w469:bool)
            "AI2 Y Sum Set 1" <- w471
            "AI1 X Set 1" <- w470
          }
          frame 2 {
            n221 = Unbundle By Name(w483) -> ("Set 2"=w482:bool)
            n222 = local read "BD1 Frequency Out 2"() -> (w477:u64)
            n223 = Compound Arithmetic op=AND(w480, w482, w481) -> (w476:bool)
            "AI2 Y Sum Set 2" <- w479
            "AI1 X Set 2" <- w478
          }
          frame 3 {
            n224 = Unbundle By Name(w489) -> ("Set 3"=w488:bool)
          }
        }
        n225 = And(x=w438, y=w432) -> (x .and. y?=w440:bool)
        n226 = case shown="True" w440 {
          tunnel: w449 -> [_ w503]
          tunnel: w413 -> [_ w502]
          tunnel: w414 -> [_ w501]
          tunnel: w448 -> [_ w500]
          tunnel: w437 -> [_ w499]
          tunnel: w436 -> [_ w498]
          tunnel: w435 -> [_ w497]
          tunnel: w434 -> [_ w496]
          tunnel: 0 ("DMA buffer timeout") -> [_ w505]
          frame False {
          }
          frame True {
            n227 = Build Array(w503, w502, w501, w500, w499, w498, w497, w496) -> (w504:void[])
            n228 = for {
              tunnel: w504 -> [w507] mode=indexing
              tunnel: w505 -> [w508]
              tunnel: [w506] -> w494 mode=indexing
              n229 = xnode ("FIFO Write")("Element"=w507, "Timeout"=w508) -> ("Timed Out?"=w506:bool)  [unwired: 1 in, 1 out]
            }
            n230 = Or Array Elements(Boolean array=w494) -> (logical OR=w491:bool)
            n231 = Boolean To (0,1)(Boolean=w491) -> (0, 1=w493:i16)
            n232 = feedback #23(u16 0) -> (w492:u16)
            n233 = Add(x=w493, y=w492) -> (x+y=w490:u16)
            "Trap AI FIFO Timeout" <- w490
            n234 = feedback-in #23(w490) -> ()
          }
        }
        n235 = feedback-in #21(w416) -> ()
        n236 = feedback-in #22(w432) -> ()
        n237 = case shown="True" w397 {
          tunnel: w396 -> [_ w455]
          tunnel: [u8 0 w452] -> w395
          frame False {
          }
          frame True {
            n238 = Split Number(x=w455) -> (hi(x)=w456:u32, lo(x)=w457:u32)
            n239 = Split Number(x=w456) -> (lo(x)=w458:u16)  [unwired: 1 out]
            n240 = Split Number(x=w457) -> (hi(x)=w459:u16, lo(x)=w460:u16)
            n241 = Build Array "BD 1 nu Stack"(w458, w459, w460) -> (w454:u16[])
            n242 = for {
              tunnel: w454 -> [w467] mode=indexing
              shift-right: [w463] -> w452
              shift-left: u8 0 -> [w464]
              n243 = xnode ("FIFO Method Node")("Element"=w467, "Timeout"="Trap FIFO Set Timeout") -> ("Timed Out?"=w466:bool)  [unwired: 1 in, 1 out]
              n244 = Boolean To (0,1)(Boolean=w466) -> (0, 1=w465:i16)
              n245 = To Unsigned Byte Integer(number=w465) -> (unsigned 8bit integer=w462:u8)
              n246 = Add(x=w462, y=w464) -> (x+y=w463:u8)
            }
          }
        }
        n247 = To Unsigned Word Integer(number=w395) -> (unsigned 16bit integer=w394:u16)
        n248 = feedback #24(u16 0) -> (w408:u16)
        n249 = Add(x=w394, y=w408) -> (x+y=w407:u16)
        "Trap Pos FIFO Timeout" <- w407
        n250 = feedback-in #24(w407) -> ()
        n251 = feedback-in #25(w431) -> ()
        n252 = feedback #25(w431) -> (w430:u16)
        n253 = Subtract(x=w431, y=w430) -> (x-y=w429:u16)
        n254 = xnode "FPGA I/O Node"("Connector1/DIO31"=FALSE ("Connector1/DIO34")) -> ()  [unwired: 1 in, 1 out]
        n255 = Subtract(x=w429, y=w428) -> (x-y=w399:u16)
        n256 = Boolean To (0,1)(Boolean="+ phase") -> (0, 1=w424:i16)
        n257 = Multiply(x=w424, y="Phase count adjustment") -> (x*y=w418:i16)
        n258 = Subtract(x="ai count", y=w399) -> (x-y=w422:u16)
        n259 = Number To Boolean Array(number=w399) -> (Boolean array=w400:bool[])
        n260 = feedback #26(i16 0) -> (w420:i16)
        n261 = Add(x=w422, y=w418) -> (x+y=w421:u16)
        n262 = Subtract(x=w420, y=w418) -> (x-y=w419:i16)
        "Relative phase" <- w419
        n263 = feedback-in #26(w419) -> ()
        n264 = Or Array Elements(Boolean array=w400) -> (logical OR=w398:bool)
        n265 = Boolean To (0,1)(Boolean=w398) -> (0, 1=w405:i16)
        n266 = To Unsigned Byte Integer(number=w405) -> (unsigned 8bit integer=w402:u8)
        n267 = feedback #27(u8 0) -> (w403:u8)
        n268 = Add(x=w402, y=w403) -> (x+y=w401:u8)
        "AI Late Counter" <- w401
        n269 = feedback-in #27(w401) -> ()
      }
    }
  }
  n270 = while "MCL stage control" {
    shift-right: [w524] -> _
    shift-left: w3 -> [w527]
    shift-right: [w517] -> _
    shift-left: w8 -> [w514]
    shift-right: [w516] -> _
    shift-left: w7 -> [w512]
    i -> [w511]
    stop <- FALSE stop-if-true
    n271 = flat-sequence {
      tunnel: w527 -> [w531]
      tunnel: [w532] -> w523
      tunnel: [w531] -> w521
      tunnel: [w530] -> w515
      tunnel: w514 -> [w530]
      tunnel: [w529] -> w513
      tunnel: w512 -> [w529]
      tunnel: w523 -> [w536]
      tunnel: [w536] -> w522
      tunnel: w521 -> [w535]
      tunnel: [w535] -> w520
      tunnel: w515 -> [w534]
      tunnel: w513 -> [w533]
      tunnel: [w534] -> w510
      tunnel: [w533] -> w509
      tunnel: w522 -> [w546]
      tunnel: w520 -> [w545]
      tunnel: [w546] -> w526
      tunnel: [w545] -> w525
      tunnel: [w544] -> w519
      tunnel: [w543] -> w518
      tunnel: w510 -> [w538]
      tunnel: w509 -> [w537]
      tunnel: [w618] -> w524
      tunnel: w526 -> [w625]
      tunnel: w525 -> [w622]
      tunnel: w519 -> [w620]
      tunnel: w518 -> [w619]
      tunnel: [w620] -> w517
      tunnel: [w619] -> w516
      frame #0 {
        n272 = call "Loop Timer5"("Count(Ticks)"=w531) -> ("Tick Count(Ticks)"=w532:u32)
      }
      frame #1 {
        n273 = xnode "FPGA I/O Node"("Connector0/AO1"=w534, "Connector0/AO2"=w533) -> ()  [unwired: 2 in, 2 out]
      }
      frame #2 {
        n274 = local read "Scanning MCL"() -> (w558:bool)
        n275 = Or(x=w558, y="Start scan (MCL)") -> (x .or. y?=w553:bool)
        n276 = Not(x="Abort scan (MCL)") -> (.not. x?=w551:bool)
        n277 = And(x=w551, y=w553) -> (x .and. y?=w550:bool)
        n278 = case "Raster scan" shown="True" w550 {
          tunnel: [w559 w602] -> w555
          tunnel: "Start scan (MCL)" -> [_ w587]
          tunnel: [w559 w563] -> w539
          frame False {
            w559 = i16 0
            n279 = local write "Scanning MCL"(FALSE ("scanning")) -> ()
          }
          frame True {
            w573 = i16 0
            w572 = u64 0
            # "scan incr."
            # "freq. incr. mult."
            # "count steps"
            # "count number of cycles"
            n280 = feedback #28(w572) -> (w599:u64)
            n281 = Select(t=w572, s=w587, f=w599) -> (s? t:f=w601:u64)
            n282 = Increment(x=w601) -> (x+1=w598:u64)
            n283 = Greater?(x="Cycles per step (MCL)", y=w598) -> (0:w582:bool)
            n284 = Select(t=w598, s=w582, f=w572) -> (s? t:f=w597:u64)
            n285 = feedback-in #28(w597) -> ()
            n286 = feedback #29(w572) -> (w596:u64)
            n287 = Select(t=w572, s=w587, f=w596) -> (s? t:f=w591:u64)
            n288 = Increment(x=w591) -> (x+1=w595:u64)
            n289 = Add(x="Scan steps (MCL)", y="Scan steps (MCL)") -> (x+y=w594:u64)
            n290 = Select(t=w591, s=w582, f=w595) -> (s? t:f=w577:u64)
            n291 = Greater?(x=w594, y=w577) -> (0:w576:bool)
            n292 = Select(t=w577, s=w576, f=w572) -> (s? t:f=w592:u64)
            n293 = feedback-in #29(w592) -> ()
            n294 = Equal?(x="Scan steps (MCL)", y=w577) -> (x = y?=w581:bool)
            n295 = Greater?(x="Scan steps (MCL)", y=w591) -> (0:w590:bool)
            n296 = feedback #30(w573) -> (w593:i16)
            n297 = Select(t=w573, s=w587, f=w593) -> (s? t:f=w579:i16)
            n298 = Increment(x=w579) -> (x+1=w589:i16)
            n299 = Decrement(x=w579) -> (x-1=w588:i16)
            n300 = Select(t=w589, s=w590, f=w588) -> (s? t:f=w580:i16)
            n301 = Select(t=w579, s=w581, f=w580) -> (s? t:f=w578:i16)
            n302 = Select(t=w579, s=w582, f=w578) -> (s? t:f=w574:i16)
            n303 = Select(t=w574, s=w576, f=w573) -> (s? t:f=w575:i16)
            n304 = feedback-in #30(w575) -> ()
            n305 = feedback #31(w572) -> (w586:u64)
            n306 = Select(t=w572, s=w587, f=w586) -> (s? t:f=w561:u64)
            n307 = Increment(x=w561) -> (x+1=w583:u64)
            n308 = Select(t=w561, s=w576, f=w583) -> (s? t:f=w562:u64)
            n309 = Greater?(x="Number of scans (MCL)", y=w562) -> (0:w569:bool)
            n310 = Multiply(x="Scan freq.  increment (MCL)", y=w579) -> (x*y=w602:i16)
            n311 = Select(t=TRUE, s="Cont. Scan (MCL)", f=w569) -> (s? t:f=w568:bool)
            "Scanning MCL" <- w568
            n312 = Select(t=w562, s=w568, f=w572) -> (s? t:f=w584:u64)
            n313 = feedback-in #31(w584) -> ()
            n314 = Increment(x=w562) -> (x+1=→"Scan I (MCL)":u64)
            n315 = To Word Integer(number=w561) -> (16bit integer=w564:i16)
            n316 = Multiply(x=w564, y="Scan freq.  increment (MCL)") -> (x*y=w563:i16)
          }
        }
        n317 = Select(t=w539, s="1D or 2D Scan?", f=i16 0) -> (s? t:f=w540:i16)
        n318 = Select(t=w540, s="MCL Scan Axis", f=w555) -> (s? t:f=w554:i16)
        n319 = Select(t=w555, s="MCL Scan Axis", f=w540) -> (s? t:f=w556:i16)
        n320 = Add(x=w554, y="AO2") -> (x+y=w543:i16)
        n321 = Add(x="AO1", y=w556) -> (x+y=w544:i16)
        "AO1 2" <- w538
        "AO2 2" <- w537
      }
      frame #3 {
        n322 = feedback-in #32(w625) -> ()
        n323 = feedback #32(w625) -> (w624:u32)
        n324 = Boolean To (0,1)(Boolean="+ phase (MCL)") -> (0, 1=w616:i16)
        n325 = Subtract(x=w625, y=w624) -> (x-y=w623:u32)
        n326 = Multiply(x=w616, y="Phase count adjustment (MCL)") -> (x*y=w612:i16)
        n327 = Subtract(x=w623, y=w622) -> (x-y=w604:u32)
        n328 = Subtract(x="MCL count", y=w604) -> (x-y=w614:u32)
        n329 = feedback #33(i16 0) -> (w613:i16)
        n330 = Subtract(x=w613, y=w612) -> (x-y=w611:i16)
        "MCL Relative Phase" <- w611
        n331 = feedback-in #33(w611) -> ()
        n332 = Number To Boolean Array(number=w604) -> (Boolean array=w605:bool[])
        n333 = Or Array Elements(Boolean array=w605) -> (logical OR=w603:bool)
        n334 = Boolean To (0,1)(Boolean=w603) -> (0, 1=w610:i16)
        n335 = Add(x=w614, y=w612) -> (x+y=w618:u32)
        n336 = To Unsigned Byte Integer(number=w610) -> (unsigned 8bit integer=w607:u8)
        n337 = feedback #34(u8 0) -> (w608:u8)
        n338 = Add(x=w607, y=w608) -> (x+y=w606:u8)
        "MCL Late Counter" <- w606
        n339 = feedback-in #34(w606) -> ()
      }
    }
    "Numeric" <- w511
  }
  n340 = while "RF box board direct communication loop" {
    tunnel: w3 -> [_]
    stop <- FALSE stop-if-true
    n341 = case "Whether to use direct communication method (only use one method at a time)" shown="True" "Direct RF Box \nCommunication" {
      frame False {
      }
      frame True {
        n342 = case shown="True" "Update Data" {
          frame False {
          }
          frame True {
            n343 = flat-sequence {
              frame #0 {
                n344 = First Call?() -> (First Call?: T/F=w630:bool)
                n345 = case shown="True" w630 {
                  frame False {
                  }
                  frame True {
                    # "If first time data updated, be sure to set WR high\nbefore setting data and address bits."
                    n346 = flat-sequence {
                      frame #0 {
                        n347 = xnode "FPGA I/O Node"("Connector1/DIO15"=TRUE) -> ()  [unwired: 1 in, 1 out]
                      }
                      frame #1 {
                        n348 = call "Wait"("Count(Ticks)"=u8 40 ("DO Delay 3 (Ticks)")) -> ()  [unwired: 1 out]
                      }
                    }
                  }
                }
              }
              frame #1 {
                n349 = Number To Boolean Array(number="Address") -> (Boolean array=w679:bool[])
                n350 = Number To Boolean Array(number="Data BD 1") -> (Boolean array=w680:bool[])
                n351 = Number To Boolean Array(number="Data BD 2") -> (Boolean array=w649:bool[])
                n352 = Index Array(array=w680, index=7) -> (element=w664:bool)
                n353 = Index Array(array=w680, index=6) -> (element=w663:bool)
                n354 = Index Array(array=w680, index=5) -> (element=w662:bool)
                n355 = Index Array(array=w680, index=4) -> (element=w661:bool)
                n356 = Index Array(array=w680, index=3) -> (element=w660:bool)
                n357 = Index Array(array=w680, index=2) -> (element=w659:bool)
                n358 = Index Array(array=w680, index=1) -> (element=w658:bool)
                n359 = Index Array(array=w680, index=0) -> (element=w657:bool)
                n360 = Index Array(array=w679, index=5) -> (element=w656:bool)
                n361 = Index Array(array=w679, index=4) -> (element=w655:bool)
                n362 = Index Array(array=w679, index=3) -> (element=w654:bool)
                n363 = Index Array(array=w679, index=2) -> (element=w653:bool)
                n364 = Index Array(array=w679, index=1) -> (element=w652:bool)
                n365 = Index Array(array=w679, index=0) -> (element=w651:bool)
                n366 = Index Array(array=w649, index=7) -> (element=w640:bool)
                n367 = Index Array(array=w649, index=6) -> (element=w639:bool)
                n368 = Index Array(array=w649, index=5) -> (element=w638:bool)
                n369 = Index Array(array=w649, index=4) -> (element=w637:bool)
                n370 = Index Array(array=w649, index=3) -> (element=w636:bool)
                n371 = Index Array(array=w649, index=2) -> (element=w635:bool)
                n372 = Index Array(array=w649, index=1) -> (element=w634:bool)
                n373 = Index Array(array=w649, index=0) -> (element=w633:bool)
                n374 = xnode "FPGA I/O Node"("Connector1/DIO0"=w664, "Connector1/DIO1"=w663, "Connector1/DIO2"=w662, "Connector1/DIO3"=w661, "Connector1/DIO4"=w660, "Connector1/DIO5"=w659, "Connector1/DIO6"=w658, "Connector1/DIO7"=w657, "Connector1/DIO8"=w656, "Connector1/DIO9"=w655, "Connector1/DIO10"=w654, "Connector1/DIO11"=w653, "Connector1/DIO12"=w652, "Connector1/DIO13"=w651, "Connector1/DIO20"=w640, "Connector1/DIO21"=w639, "Connector1/DIO22"=w638, "Connector1/DIO23"=w637, "Connector1/DIO24"=w636, "Connector1/DIO25"=w635, "Connector1/DIO26"=w634, "Connector1/DIO27"=w633) -> ()  [unwired: 22 in, 22 out]
              }
              frame #2 {
                # "wait and then apply write signal"
                n375 = call "Wait2"("Count(Ticks)"=u8 40 ("DO Delay 1 (Ticks)")) -> ()  [unwired: 1 out]
              }
              frame #3 {
                # "sending bit low writes data to board buffer"
                n376 = xnode "FPGA I/O Node"("Connector1/DIO15"=FALSE) -> ()  [unwired: 1 in, 1 out]
              }
              frame #4 {
                # "wait then return write signal"
                n377 = call "Wait3"("Count(Ticks)"=u8 40 ("DO Delay 2 (Ticks)")) -> ()  [unwired: 1 out]
              }
              frame #5 {
                # "sending bit high makes ready to\nwrite more data"
                n378 = xnode "FPGA I/O Node"("Connector1/DIO15"=TRUE) -> ()  [unwired: 1 in, 1 out]
              }
            }
          }
        }
      }
    }
  }
  n379 = while "Control APD data integration - stream to host" {
    shift-right: [w689] -> _
    shift-left: w3 -> [w694]
    stop <- FALSE stop-if-true
    n380 = flat-sequence {
      tunnel: w694 -> [w696]
      tunnel: [w697] -> w692
      tunnel: [w696] -> w690
      tunnel: [w705] -> w693
      tunnel: w692 -> [w705]
      tunnel: [w704] -> w691
      tunnel: w690 -> [w704]
      tunnel: [w703] -> w688
      tunnel: [w702] -> w687
      tunnel: [w739] -> w689
      tunnel: w693 -> [w751]
      tunnel: w691 -> [w748]
      tunnel: w688 -> [w732]
      tunnel: w687 -> [w731]
      frame #0 {
        n381 = call "Loop Timer6"("Count(Ticks)"=w696) -> ("Tick Count(Ticks)"=w697:u32)
      }
      frame #1 {
        n382 = flat-sequence {
          tunnel: [w707] -> w701
          tunnel: w701 -> [w709]
          tunnel: [w711] -> w700
          tunnel: [w710] -> w699
          tunnel: [w709] -> w698
          tunnel: [w717] -> w702
          tunnel: [w718] -> w703
          tunnel: w700 -> [w718]
          tunnel: w699 -> [w717]
          tunnel: w698 -> [w716]
          frame #0 {
            # "use two separate variable so each APD won't\nhave to wait to read"
            n383 = feedback #35(FALSE) -> (w706:bool)
            "APD 1 out state" <- w706
            "APD 2 out state" <- w706
            n384 = Not(x=w706) -> (.not. x?=w707:bool)
            n385 = feedback-in #35(w707) -> ()
          }
          frame #1 {
            n386 = local read "APD 1 Counts 1"() -> (w715:u32)
            n387 = local read "APD 1 Counts 0"() -> (w714:u32)
            n388 = local read "APD 2 Counts 1"() -> (w713:u32)
            n389 = local read "APD 2 Counts 0"() -> (w712:u32)
            n390 = Select(t=w715, s=w709, f=w714) -> (s? t:f=w711:u32)
            n391 = Select(t=w713, s=w709, f=w712) -> (s? t:f=w710:u32)
          }
          frame #2 {
            n392 = case shown="True" w716 {
              frame False {
                w719 = u32 0 ("APD 1 Counts 0")
                n393 = local write "APD 1 Counts 0"(w719) -> ()
                n394 = local write "APD 2 Counts 0"(w719) -> ()
              }
              frame True {
                w720 = u32 0 ("APD 1 Counts 1")
                n395 = local write "APD 1 Counts 1"(w720) -> ()
                n396 = local write "APD 2 Counts 1"(w720) -> ()
              }
            }
          }
        }
      }
      frame #2 {
        n397 = feedback-in #36(w751) -> ()
        n398 = feedback #36(w751) -> (w750:u32)
        n399 = Subtract(x=w751, y=w750) -> (x-y=w749:u32)
        n400 = Subtract(x=w749, y=w748) -> (x-y=w724:u32)
        n401 = case shown="True" "APD to FIFO" {
          tunnel: w732 -> [_ w754]
          tunnel: w731 -> [_ w752]
          frame False {
          }
          frame True {
            n402 = flat-sequence {
              tunnel: 0 ("Timeout") -> [w756]
              tunnel: w754 -> [w757]
              tunnel: [w756] -> w753
              tunnel: w753 -> [w759]
              tunnel: w752 -> [w758]
              frame #0 {
                n403 = xnode ("FIFO Write")("Element"=w757, "Timeout"=w756) -> ()  [unwired: 1 in, 2 out]
              }
              frame #1 {
                n404 = xnode ("FIFO Write")("Element"=w758, "Timeout"=w759) -> ()  [unwired: 1 in, 2 out]
              }
            }
          }
        }
        n405 = Subtract(x="APD Acq Rate Count", y=w724) -> (x-y=w740:u32)
        n406 = Number To Boolean Array(number=w724) -> (Boolean array=w725:bool[])
        n407 = Or Array Elements(Boolean array=w725) -> (logical OR=w723:bool)
        n408 = Boolean To (0,1)(Boolean=w723) -> (0, 1=w730:i16)
        n409 = To Unsigned Byte Integer(number=w730) -> (unsigned 8bit integer=w727:u8)
        n410 = Boolean To (0,1)(Boolean="+ phase (APD Acq)") -> (0, 1=w736:i16)
        n411 = feedback #37(u8 0) -> (w728:u8)
        n412 = Add(x=w727, y=w728) -> (x+y=w726:u8)
        "APD Acq Late Counter" <- w726
        n413 = feedback-in #37(w726) -> ()
        n414 = Multiply(x=w736, y="Phase Count Adjustment (APD Acq)") -> (x*y=w733:i16)
        n415 = Add(x=w740, y=w733) -> (x+y=w739:u32)
        n416 = feedback #38(i16 0) -> (w738:i16)
        n417 = Subtract(x=w738, y=w733) -> (x-y=w735:i16)
        "APD Acq Relative Phase" <- w735
        n418 = feedback-in #38(w735) -> ()
        n419 = To Word Integer(number=w732) -> (16bit integer=w741:i16)
        n420 = To Word Integer(number=w731) -> (16bit integer=w742:i16)
        n421 = Multiply(x="APD 1 AO scale factor", y=w741) -> (x*y=w722:i16)
        n422 = Multiply(x="APD 2 AO scale factor", y=w742) -> (x*y=w721:i16)
        n423 = xnode "FPGA I/O Node"("Connector0/AO5"=w722, "Connector0/AO7"=w721) -> ()  [unwired: 2 in, 2 out]
      }
    }
  }
  n424 = while "RF box board DIO control: parallel communication" {
    shift-right: [w766] -> _
    shift-left: w3 -> [w765]
    shift-right: [w764] -> _
    shift-left: FALSE ("Swap F1 and F2") -> [w763]
    stop <- FALSE stop-if-true
    n425 = flat-sequence {
      tunnel: w763 -> [w770]
      tunnel: w765 -> [w768]
      tunnel: [w770] -> w762
      tunnel: [w769] -> w761
      tunnel: [w768] -> w760
      tunnel: [w776] -> w766
      tunnel: [w775] -> w764
      tunnel: w762 -> [w774]
      tunnel: w761 -> [w772]
      tunnel: w760 -> [w771]
      frame #0 {
        n426 = call "Loop Timer"("Count(Ticks)"=w768) -> ("Tick Count(Ticks)"=w769:u16)
      }
      frame #1 {
        n427 = flat-sequence {
          tunnel: ["FPGA Controls\n RF Box"] -> w773
          tunnel: w774 -> [w777]
          tunnel: [w817] -> w776
          tunnel: [w830] -> w775
          tunnel: w773 -> [w829]
          tunnel: w772 -> [w823]
          tunnel: w771 -> [w820]
          frame #0 {
            n428 = case shown="True" "FPGA Controls\n RF Box" {
              tunnel: w777 -> [_ w779]
              frame False {
              }
              frame True {
                n429 = flat-sequence {
                  tunnel: w779 -> [w785]
                  frame #0 {
                    n430 = First Call?() -> (First Call?: T/F=w780:bool)
                    n431 = case shown="True" w780 {
                      frame False {
                      }
                      frame True {
                        # "If first time data updated, be sure to set WR high and UDCLK low\nbefore setting data and address bits."
                        n432 = xnode "FPGA I/O Method Node"("Enable"=TRUE) -> ("FPGA I/O Out"=w782:refnum<k21>)  [unwired: 1 in]
                        n433 = xnode "FPGA I/O Node"("Connector1/DIO15"=TRUE) -> ()  [unwired: 1 in, 1 out]
                        n434 = xnode "FPGA I/O Node"("I/O Item"=FALSE ("Connector1/DIO30"), "FPGA I/O In"=w782) -> ()  [unwired: 1 out]
                      }
                    }
                  }
                  frame #1 {
                    n435 = case shown="True" "Freq or Amp switch first" {
                      tunnel: w785 -> [w787 w792]
                      frame False {
                        n436 = flat-sequence {
                          tunnel: w787 -> [w791]
                          frame #0 {
                            # "switch amplitude"
                            # "send udclk high"
                            n437 = xnode "FPGA I/O Node"("Connector1/DIO30"=TRUE ("Connector1/DIO15")) -> ()  [unwired: 1 in, 1 out]
                          }
                          frame #1 {
                            # "send udclk low"
                            n438 = xnode "FPGA I/O Node"("Connector1/DIO30"=FALSE ("Connector1/DIO15")) -> ()  [unwired: 1 in, 1 out]
                          }
                          frame #2 {
                            n439 = call "Wait5"("Count(Ticks)"="Freq switch delay") -> ()  [unwired: 1 out]
                          }
                          frame #3 {
                            # "switch frequency"
                            n440 = xnode "FPGA I/O Node"("Connector1/DIO36"=w791) -> ()  [unwired: 1 in, 1 out]
                          }
                        }
                      }
                      frame True {
                        n441 = flat-sequence {
                          tunnel: w792 -> [w793]
                          frame #0 {
                            # "switch frequency"
                            n442 = xnode "FPGA I/O Node"("Connector1/DIO36"=w793) -> ()  [unwired: 1 in, 1 out]
                          }
                          frame #1 {
                            n443 = call "Wait4"("Count(Ticks)"="Amp switch delay") -> ()  [unwired: 1 out]
                          }
                          frame #2 {
                            # "switch amplitude"
                            # "send udclk high"
                            n444 = xnode "FPGA I/O Node"("Connector1/DIO30"=TRUE ("Connector1/DIO15")) -> ()  [unwired: 1 in, 1 out]
                          }
                          frame #3 {
                            # "send udclk low"
                            n445 = xnode "FPGA I/O Node"("Connector1/DIO30"=FALSE ("Connector1/DIO15")) -> ()  [unwired: 1 in, 1 out]
                          }
                        }
                      }
                    }
                  }
                }
              }
            }
          }
          frame #1 {
            # "This is the prior cycle's on time"
            # "increment timing\nindex, reset to 0 if \nend of matrix"
            # "Reset to begginning (1) when number of cycles reached."
            # "timing index"
            # "build byte stacks for writing data\n(must correspond to addresses array constant)"
            # "Timing housekeeping"
            # "Adjust phase if late\n(maintains constant phase relationship between cycles)"
            n446 = feedback #39(u8 0 ("t")) -> (w826:u8)
            n447 = Increment(x=w826) -> (x+1=w870:u8)
            n448 = Increment(x="Number Interlace Cycles") -> (x+1=w865:u8)
            n449 = Equal?(x=w870, y=w865) -> (x = y?=w872:bool)
            n450 = Select(t=u8 1, s=w872, f=w870) -> (s? t:f=w825:u8)
            n451 = feedback-in #39(w825) -> ()
            n452 = Increment(x=w825) -> (x+1=w867:u8)
            n453 = Equal?(x=w867, y=w865) -> (x = y?=w868:bool)
            n454 = Select(t=u8 1, s=w868, f=w867) -> (s? t:f=w864:u8)
            n455 = Select(t=w864, s="Interlace ON/OFF", f="Interlace Off Parameters") -> (s? t:f=w848:u8)
            n456 = case shown="1, Default" w848 {
              tunnel: [w942 w1107 "BD 1 Frequency 3"] -> w860
              tunnel: [w941 "BD 2 Frequency 2" "BD 2 Frequency 3"] -> w849
              tunnel: ["BD 2 Amplitude 1" "BD 2 Amplitude 2" "BD 2 Amplitude 3"] -> w805
              tunnel: [w931 w1117 "BD 1 Amplitude 3"] -> w808
              frame 1, Default {
                w922 = fxp<+/-,24,9> 0.0 ("AI1 X Set 2")
                w915 = u16 0
                w937 = u64 0 ("f")
                # "This signal integration happens no matter what\nso that correct setpoints can be chosen before \nturning on the FB."
                # "Trap 1"
                n457 = local read "AI1 X Set 2"() -> (w918:fxp<+/-,16,1>)
                n458 = local read "AI1 X Set 1"() -> (w919:fxp<+/-,16,1>)
                n459 = local read "Scanning"() -> (w943:bool)
                n460 = case shown="False" "Diff FB Measurement?" {
                  tunnel: w918 -> [w951 w960]
                  tunnel: w919 -> [w950 w961]
                  tunnel: [w948 w952] -> w920
                  frame False {
                    n461 = Select(t=w950, s="Trap Pos FB Monitor T1 or T2", f=w951) -> (s? t:f=w948:fxp<+/-,16,1>)
                  }
                  frame True {
                    n462 = Subtract(x=w961, y=w960) -> (x-y=w953:fxp<+/-,17,2>)
                    n463 = Not(x="Negate Diff?") -> (.not. x?=w959:bool)
                    n464 = Boolean To (0,1)(Boolean="Negate Diff?") -> (0, 1=w957:i16)
                    n465 = Boolean To (0,1)(Boolean=w959) -> (0, 1=w958:i16)
                    n466 = Negate(x=w957) -> (-x=w956:i16)
                    n467 = Add(x=w956, y=w958) -> (x+y=w954:i16)
                    n468 = Multiply(x=w954, y=w953) -> (x*y=w952:fxp<+/-,32,17>)
                  }
                }
                n469 = Or(x=w943, y="Start scan") -> (x .or. y?=w935:bool)
                n470 = Not(x="Abort scan") -> (.not. x?=w933:bool)
                n471 = And(x=w933, y=w935) -> (x .and. y?=w906:bool)
                n472 = feedback #40(w915) -> (w914:u16)
                n473 = Increment(x=w914) -> (x+1=w916:u16)
                n474 = Greater Or Equal?(x=w916, y="Trap Pos FB Int Count") -> (x >= y?=w907:bool)
                n475 = case "For raster scanning" shown="False" w906 {
                  tunnel: [w1048 w1060] -> w938
                  tunnel: "Start scan" -> [_ w1084]
                  frame False {
                    # "For wiggle-calibration: sinusoidal wave"
                    n476 = local read "Wiggling 1"() -> (w1043:bool)
                    n477 = Not(x="Abort wiggle 1") -> (.not. x?=w1046:bool)
                    n478 = Or(x="Wiggle trap 1", y=w1043) -> (x .or. y?=w1042:bool)
                    n479 = And(x=w1042, y=w1046) -> (x .and. y?=w1045:bool)
                    n480 = case shown="True" w1045 {
                      tunnel: [u64 0 w1056] -> w1048
                      frame False {
                        n481 = local write "Wiggling 1"(FALSE ("Wiggle")) -> ()
                      }
                      frame True {
                        # "Input is periods/tick, not Hz,\nso need to normalize by clock\nfrequency (40 MHz)."
                        n482 = Divide(x="Wiggle freq 1 (Hz)", y=fxp<+,17,26> 40000000.0) -> (x/y=w1053:fxp<+/-,17,-9>)
                        n483 = call "Sine Wave Generator"("frequency (periods/tick)"=w1053) -> ("sine out"=w1058:i32)  [unwired: 14 in]
                        n484 = Multiply(x=w1058, y="Wiggle amp 1") -> (x*y=w1056:u64)
                        "Wiggling 1" <- TRUE
                      }
                    }
                    n485 = local write "Scanning"(FALSE ("scanning")) -> ()
                  }
                  frame True {
                    w1068 = i64 0
                    w1067 = u64 0
                    # "scan incr."
                    # "freq. incr. mult."
                    # "count steps"
                    # "count number of cycles"
                    n486 = feedback #41(w1067) -> (w1096:u64)
                    n487 = Select(t=w1067, s=w1084, f=w1096) -> (s? t:f=w1098:u64)
                    n488 = Increment(x=w1098) -> (x+1=w1095:u64)
                    n489 = Greater?(x="Cycles per step", y=w1095) -> (0:w1077:bool)
                    n490 = Select(t=w1095, s=w1077, f=w1067) -> (s? t:f=w1094:u64)
                    n491 = feedback-in #41(w1094) -> ()
                    n492 = feedback #42(w1067) -> (w1093:u64)
                    n493 = Select(t=w1067, s=w1084, f=w1093) -> (s? t:f=w1088:u64)
                    n494 = Increment(x=w1088) -> (x+1=w1092:u64)
                    n495 = Add(x="Scan steps", y="Scan steps") -> (x+y=w1091:u64)
                    n496 = Select(t=w1088, s=w1077, f=w1092) -> (s? t:f=w1072:u64)
                    n497 = Greater?(x=w1091, y=w1072) -> (0:w1071:bool)
                    n498 = Select(t=w1072, s=w1071, f=w1067) -> (s? t:f=w1089:u64)
                    n499 = feedback-in #42(w1089) -> ()
                    n500 = Equal?(x="Scan steps", y=w1072) -> (x = y?=w1076:bool)
                    n501 = Greater?(x="Scan steps", y=w1088) -> (0:w1087:bool)
                    n502 = feedback #43(w1068) -> (w1090:i64)
                    n503 = Select(t=w1068, s=w1084, f=w1090) -> (s? t:f=w1074:i64)
                    n504 = Increment(x=w1074) -> (x+1=w1086:i64)
                    n505 = Decrement(x=w1074) -> (x-1=w1085:i64)
                    n506 = Select(t=w1086, s=w1087, f=w1085) -> (s? t:f=w1075:i64)
                    n507 = Select(t=w1074, s=w1076, f=w1075) -> (s? t:f=w1073:i64)
                    n508 = Select(t=w1074, s=w1077, f=w1073) -> (s? t:f=w1069:i64)
                    n509 = Select(t=w1069, s=w1071, f=w1068) -> (s? t:f=w1070:i64)
                    n510 = feedback-in #43(w1070) -> ()
                    n511 = feedback #44(w1067) -> (w1083:u64)
                    n512 = Select(t=w1067, s=w1084, f=w1083) -> (s? t:f=w1079:u64)
                    n513 = Increment(x=w1079) -> (x+1=w1080:u64)
                    n514 = Select(t=w1079, s=w1071, f=w1080) -> (s? t:f=w1078:u64)
                    n515 = Greater?(x="Number of scans", y=w1078) -> (0:w1064:bool)
                    n516 = Multiply(x="Scan freq.  increment", y=w1074) -> (x*y=w1060:i64)
                    n517 = Select(t=TRUE, s="Cont. Scan", f=w1064) -> (s? t:f=w1063:bool)
                    "Scanning" <- w1063
                    n518 = Select(t=w1078, s=w1063, f=w1067) -> (s? t:f=w1081:u64)
                    n519 = feedback-in #44(w1081) -> ()
                    n520 = Increment(x=w1078) -> (x+1=→"Scan I":u64)
                  }
                }
                n521 = Select(t=w915, s=w907, f=w916) -> (s? t:f=w917:u16)
                n522 = feedback-in #40(w917) -> ()
                n523 = feedback #45(w922) -> (w921:fxp<+/-,24,9>)
                n524 = Add(x=w920, y=w921) -> (x+y=w913:fxp<+/-,24,9>)
                n525 = Select(t=w922, s=w907, f=w913) -> (s? t:f=w925:fxp<+/-,24,9>)
                n526 = feedback-in #45(w925) -> ()
                n527 = Divide(x=w913, y="Trap Pos FB Int Count") -> (x/y=w908:fxp<+/-,16,1>)
                n528 = feedback #46(fxp<+/-,24,9> 0.0 ("AI1 X Set 2")) -> (w926:fxp<+/-,24,9>)
                n529 = Select(t=w913, s=w907, f=w926) -> (s? t:f=w927:fxp<+/-,24,9>)
                "Trap Pos FB Int Signal" <- w927
                n530 = feedback-in #46(w927) -> ()
                n531 = feedback #47(fxp<+/-,16,1> 0.0 ("Trap Pos FB Int-Norm Signal")) -> (w910:fxp<+/-,16,1>)
                n532 = Select(t=w908, s=w907, f=w910) -> (s? t:f=w909:fxp<+/-,16,1>)
                "Trap Pos FB Int-Norm Signal" <- w909
                n533 = feedback-in #47(w909) -> ()
                n534 = case "For position feedback" shown="True" "Force feedback" {
                  tunnel: [i64 0 w967] -> w928
                  tunnel: w908 -> [_ w964]
                  tunnel: w907 -> [_ w963]
                  frame False {
                  }
                  frame True {
                    n535 = feedback #48(i64 0) -> (w966:i64)
                    n536 = case shown="True" w963 {
                      tunnel: [w968 w975] -> w967
                      tunnel: w966 -> [w968 _]
                      tunnel: w964 -> [_ w969]
                      frame False {
                      }
                      frame True {
                        w979 = u32 0
                        n537 = xnode ("PID")("process variable"=w969, "reset?"="Trap Pos. FB Reset", "setpoint"="Trap Pos. FB SP", "PID gains"="Trap Pos. FB Gains", "output range"="Trap Pos. FB Range") -> ("output"=w991:fxp<+/-,16,1>)
                        n538 = Negate(x=w991) -> (-x=w990:fxp<+/-,17,2>)
                        n539 = Select(t=w990, s="Trap Pos FB Negate Action", f=w991) -> (s? t:f=w987:fxp<+/-,17,2>)
                        n540 = Scale By Power Of 2(n=u32 15, x=u32 1) -> (x*2^n=w984:u32)
                        n541 = Multiply(x=w987, y=w984) -> (x*y=w983:fxp<+/-,17,17>)
                        n542 = To Quad Integer(1:w983) -> (0:w995:i64)
                        "Trap Pos FB Action" <- w995
                        n543 = Multiply(x=w995, y="Trap Pos. FB Mult Factor") -> (x*y=w993:i64)
                        n544 = Add(x=w993, y="Trap Pos. FB Offset Factor") -> (x+y=w975:i64)
                        n545 = feedback #49() -> (w976:i64)  [unwired: 1 in]
                        n546 = Add(x=w975, y=w976) -> (x+y=w973:i64)
                        n547 = feedback #50(w979) -> (w981:u32)
                        n548 = Increment(x=w981) -> (x+1=w970:u32)
                        n549 = Greater Or Equal?(x=w970, y="FB Trig Integrate") -> (x >= y?=w971:bool)
                        n550 = Select(t=i64 0, s=w971, f=w973) -> (s? t:f=w977:i64)
                        n551 = feedback-in #49(w977) -> ()
                        n552 = Select(t=w979, s=w971, f=w970) -> (s? t:f=w980:u32)
                        n553 = feedback-in #50(w980) -> ()
                        n554 = And(x=w971, y="FPGA Trap Trig") -> (x .and. y?=w978:bool)
                        n555 = case "Trap FB trigger excitation laser ON" shown="True" w978 {
                          tunnel: w973 -> [_ w1001]
                          tunnel: w970 -> [_ w999]
                          frame False {
                          }
                          frame True {
                            n556 = Not(x="TTrig Negate Pos") -> (.not. x?=w1008:bool)
                            n557 = Boolean To (0,1)(Boolean="TTrig Negate Pos") -> (0, 1=w1006:i16)
                            n558 = Boolean To (0,1)(Boolean=w1008) -> (0, 1=w1007:i16)
                            n559 = Negate(x=w1006) -> (-x=w1005:i16)
                            n560 = Add(x=w1005, y=w1007) -> (x+y=w1004:i16)
                            n561 = Multiply(x=w1004, y=w1001) -> (x*y=w1003:i64)
                            "TTrig Sig" <- w1003
                            n562 = Multiply(x="FPGA TTrig Thresh", y=w999) -> (x*y=w1000:i64)
                            "TTrig Fin Thresh" <- w1000
                            n563 = Greater Or Equal?(x=w1003, y=w1000) -> (x >= y?=w1002:bool)
                            n564 = case shown="True" w1002 {
                              frame False {
                              }
                              frame True {
                                w1011 = TRUE ("Green FB On/Off")
                                w1013 = u8 2 ("Operating Mode")
                                n565 = local write "Operating Mode 2"(w1013) -> ()
                                n566 = local write "Operating Mode"(w1013) -> ()
                                n567 = local write "Green FB On/Off"(w1011) -> ()
                                n568 = local write "FPGA Trap Trig"(FALSE ("FPGA Trap Trig")) -> ()
                                "TTrig?" <- w1011
                              }
                            }
                          }
                        }
                      }
                    }
                    n569 = feedback-in #48(w967) -> ()
                  }
                }
                n570 = case "For intensity feedback" shown="True" "FB On/Off Set 1" {
                  tunnel: "BD 1 Amplitude 1" -> [w1099 _]
                  tunnel: [w1099 w1100] -> w931
                  frame False {
                  }
                  frame True {
                    n571 = local read "AI2 Y Sum Set 1"() -> (w1102:i16)
                    n572 = call "Slower PID.vi"("process variable"=w1102, "reset?"="FB Reset Set 1", "setpoint"="FB Setpoint Set 1", "PID gains (x 2^8)"="FB Gains Set 1", "output range"="FB output range 1") -> ("output"=w1105:i16)  [unwired: 10 out]
                    n573 = To Unsigned Word Integer(number=w1105) -> (unsigned 16bit integer=w1100:u16)
                  }
                }
                n574 = Select(t=w937, s="Scan BD", f=w938) -> (s? t:f=w936:u64)
                n575 = Select(t=w938, s="Scan BD", f=w937) -> (s? t:f=w939:u64)
                n576 = Add(x=w936, y="BD 2 Frequency 1") -> (x+y=w941:u64)
                n577 = Compound Arithmetic op=ADD("BD 1 Frequency 1", w928, w939) -> (w942:u64)
                "BD1 Frequency Out 1" <- w942
              }
              frame 2 {
                # "For wiggle calibration"
                # "Trap 2"
                n578 = local read "Wiggling 2"() -> (w1114:bool)
                n579 = Or(x="Wiggle trap 2", y=w1114) -> (x .or. y?=w1113:bool)
                n580 = Not(x="Abort wiggle 2") -> (.not. x?=w1111:bool)
                n581 = And(x=w1113, y=w1111) -> (x .and. y?=w1110:bool)
                n582 = case shown="True" "FB On/Off Set 2" {
                  tunnel: [w1130 w1131] -> w1117
                  tunnel: "BD 1 Amplitude 2" -> [w1130 _]
                  frame False {
                  }
                  frame True {
                    n583 = local read "AI2 Y Sum Set 2"() -> (w1136:i16)
                    n584 = call "Slower PID.vi"("process variable"=w1136, "reset?"="FB Reset Set 2", "setpoint"="FB Setpoint Set 2", "PID gains (x 2^8)"="FB Gains Set 2", "output range"="FB output range 2") -> ("output"=w1133:i16)  [unwired: 10 out]
                    n585 = To Unsigned Word Integer(number=w1133) -> (unsigned 16bit integer=w1131:u16)
                  }
                }
                n586 = case shown="True" w1110 {
                  tunnel: [i16 0 w1124] -> w1108
                  frame False {
                    n587 = local write "Wiggling 2"(FALSE) -> ()
                  }
                  frame True {
                    n588 = Divide(x="Wiggle freq 2 (Hz)", y=fxp<+,17,26> 40000000.0) -> (x/y=w1127:fxp<+/-,17,-9>)
                    n589 = call "Sine Wave Generator2"("frequency (periods/tick)"=w1127) -> ("sine out"=w1126:i32)  [unwired: 14 in]
                    n590 = Multiply(x=w1126, y="Wiggle amp 2") -> (x*y=w1124:u64)
                    "Wiggling 2" <- TRUE
                  }
                }
                n591 = Add(x="BD 1 Frequency 2", y=w1108) -> (x+y=w1107:u64)
                "BD1 Frequency Out 2" <- w1107
              }
              frame 3 {
                # "Fluorescence period"
              }
            }
            n592 = feedback-in #51(w823) -> ()
            n593 = feedback #51(w823) -> (w822:u16)
            n594 = Select(t=w825, s="Interlace ON/OFF", f="Interlace Off Parameters") -> (s? t:f=w863:u8)
            n595 = Subtract(x=w823, y=w822) -> (x-y=w821:u16)
            n596 = Subtract "The error"(x=w821, y=w820) -> (x-y=w798:u16)
            n597 = case shown="3" w863 {
              tunnel: ["DIO count 1 (ticks)" "DIO count 2 (ticks)" "DIO count 3 (ticks)"] -> w819
              frame 1, Default {
              }
              frame 2 {
              }
              frame 3 {
              }
            }
            n598 = Number To Boolean Array(number=w798) -> (Boolean array=w799:bool[])
            n599 = Or Array Elements(Boolean array=w799) -> (logical OR=w797:bool)
            n600 = Boolean To (0,1)(Boolean=w797) -> (0, 1=w804:i16)
            n601 = To Unsigned Byte Integer(number=w804) -> (unsigned 8bit integer=w801:u8)
            n602 = feedback #52(u8 0) -> (w802:u8)
            n603 = Add(x=w801, y=w802) -> (x+y=w800:u8)
            "DIO Late Counter" <- w800
            n604 = feedback-in #52(w800) -> ()
            n605 = Subtract(x=w819, y=w798) -> (x-y=w818:u16)
            n606 = Split Number(x=w860) -> (hi(x)=w859:u32, lo(x)=w858:u32)
            n607 = Split Number(x=w849) -> (hi(x)=w854:u32, lo(x)=w853:u32)
            n608 = Boolean To (0,1)(Boolean="+ phase (DIO)") -> (0, 1=w815:i16)
            n609 = Split Number(x=w859) -> (lo(x)=w857:u16)  [unwired: 1 out]
            n610 = Split Number(x=w858) -> (hi(x)=w856:u16, lo(x)=w855:u16)
            n611 = Split Number(x=w854) -> (lo(x)=w852:u16)  [unwired: 1 out]
            n612 = Split Number(x=w853) -> (hi(x)=w851:u16, lo(x)=w850:u16)
            n613 = Split Number(x=w808) -> (hi(x)=w810:u8, lo(x)=w809:u8)
            n614 = Split Number(x=w805) -> (hi(x)=w807:u8, lo(x)=w806:u8)
            n615 = Split Number(x=w857) -> (hi(x)=w847:u8, lo(x)=w846:u8)
            n616 = Split Number(x=w856) -> (hi(x)=w845:u8, lo(x)=w844:u8)
            n617 = Split Number(x=w852) -> (hi(x)=w840:u8, lo(x)=w839:u8)
            n618 = Split Number(x=w855) -> (hi(x)=w843:u8, lo(x)=w842:u8)
            n619 = Split Number(x=w851) -> (hi(x)=w838:u8, lo(x)=w837:u8)
            n620 = Split Number(x=w850) -> (hi(x)=w836:u8, lo(x)=w835:u8)
            n621 = Multiply(x=w815, y="Phase count adjustment (DIO)") -> (x*y=w811:i16)
            n622 = feedback #53(i16 0) -> (w813:i16)
            n623 = Subtract(x=w813, y=w811) -> (x-y=w812:i16)
            "DIO Relative phase" <- w812
            n624 = feedback-in #53(w812) -> ()
            n625 = Add(x=w818, y=w811) -> (x+y=w817:u16)
            n626 = Build Array "BD 1 A Stack"(w810, w809) -> (w832:u8[])
            n627 = Build Array "BD 2 A Stack"(w807, w806) -> (w831:u8[])
            n628 = Build Array "BD 1 nu Stack"(w847, w846, w845, w844, w843, w842) -> (w841:u8[])
            n629 = Build Array "BD 2 nu Stack"(w840, w839, w838, w837, w836, w835) -> (w834:u8[])
            n630 = case shown="2" w848 {
              tunnel: [w898 w901] -> w830
              tunnel: [u8 10 u8 4] -> w833
              tunnel: "Swap F1 and F2" -> [w899 w901]
              frame 2 {
                # "F2"
                n631 = Not(x=w899) -> (.not. x?=w898:bool)
              }
              frame 1, Default {
                # "low chooses F1"
                # "F1"
              }
            }
            n632 = case "If FPGA is controlling (toggling) RF synth" shown="True" w829 {
              tunnel: w841 -> [_ w877]
              tunnel: w834 -> [_ w876]
              tunnel: w833 -> [_ w875]
              tunnel: w832 -> [_ w874]
              tunnel: w831 -> [_ w873]
              frame False {
              }
              frame True {
                # "Write next amp.\n(wait until beginning of next loop iteration to update)"
                n633 = flat-sequence "Update the next F1 and F2 frequency value (the actual frequency won't change until FSK is switched).\nThen load the next amplitude value into buffer, but don't update it until the next cycle." {
                  tunnel: w877 -> [w880]
                  tunnel: w876 -> [w879]
                  tunnel: w875 -> [w878]
                  tunnel: w874 -> [w891]
                  tunnel: w873 -> [w890]
                  frame #0 {
                    n634 = for {
                      tunnel: w880 -> [w886] mode=indexing
                      tunnel: w879 -> [w885] mode=indexing
                      tunnel: w878 -> [w883]
                      i -> [w884]
                      # "Write next freq."
                      n635 = To Unsigned Byte Integer(number=w884) -> (unsigned 8bit integer=w881:u8)
                      n636 = Add(x=w883, y=w881) -> (x+y=w882:u8)
                      n637 = call "write to RF synth bd.vi"("Address Byte"=w882, "BD 2 Byte"=w885, "BD 1 Byte"=w886) -> ()
                    }
                  }
                  frame #1 {
                    # "send udclk high"
                    n638 = xnode "FPGA I/O Node"("Connector1/DIO30"=TRUE ("Connector1/DIO15")) -> ()  [unwired: 1 in, 1 out]
                  }
                  frame #2 {
                    n639 = xnode "FPGA I/O Node"("Connector1/DIO30"=FALSE ("Connector1/DIO15")) -> ()  [unwired: 1 in, 1 out]
                  }
                  frame #3 {
                    n640 = for {
                      tunnel: w891 -> [w897] mode=indexing
                      tunnel: w890 -> [w896] mode=indexing
                      tunnel: u8 33 -> [w894]
                      i -> [w895]
                      n641 = To Unsigned Byte Integer(number=w895) -> (unsigned 8bit integer=w892:u8)
                      n642 = Add(x=w894, y=w892) -> (x+y=w893:u8)
                      n643 = call "write to RF synth bd.vi"("Address Byte"=w893, "BD 2 Byte"=w896, "BD 1 Byte"=w897) -> ()
                    }
                  }
                }
              }
            }
          }
        }
      }
    }
  }
  n644 = node-c288(w5) -> ()
  n645 = while {
    shift-right: [w1147] -> _
    shift-left: w2 -> [w1149]
    shift-right: [w1142] -> _
    shift-left: w3 -> [w1151]
    stop <- FALSE stop-if-true
    n646 = flat-sequence {
      tunnel: w1151 -> [w1152]
      tunnel: [w1154] -> w1150
      tunnel: w1149 -> [w1154]
      tunnel: [w1153] -> w1145
      tunnel: [w1152] -> w1143
      tunnel: w1150 -> [w1157]
      tunnel: [w1156] -> w1146
      tunnel: w1145 -> [w1156]
      tunnel: [w1155] -> w1144
      tunnel: w1143 -> [w1155]
      tunnel: [w1185] -> w1147
      tunnel: w1146 -> [w1175]
      tunnel: w1144 -> [w1174]
      tunnel: [w1158] -> w1142
      frame #0 {
        n647 = call "Loop Timer11"("Count(Ticks)"=w1152) -> ("Tick Count(Ticks)"=w1153:u16)
      }
      frame #1 {
        n648 = xnode "FPGA I/O Node"("Connector1/DIO32"=w1157, "Connector1/DIO33"=w1157, "Connector1/DIO34"=w1157) -> ()  [unwired: 3 in, 3 out]
      }
      frame #2 {
        n649 = feedback #54(w1175) -> (w1184:u16)
        n650 = feedback-in #54(w1175) -> ()
        n651 = Subtract(x=w1175, y=w1184) -> (x-y=w1183:u16)
        n652 = Subtract(x=w1183, y=w1174) -> (x-y=w1170:u16)
        n653 = Number To Boolean Array(number=w1170) -> (Boolean array=w1177:bool[])
        n654 = Boolean To (0,1)(Boolean="+ phase (RI)") -> (0, 1=w1168:i16)
        n655 = Or Array Elements(Boolean array=w1177) -> (logical OR=w1176:bool)
        n656 = Multiply(x=w1168, y="Phase count adjustment (RI)") -> (x*y=w1166:i16)
        n657 = Boolean To (0,1)(Boolean=w1176) -> (0, 1=w1182:i16)
        n658 = feedback #55(i16 0) -> (w1167:i16)
        n659 = Subtract(x=w1167, y=w1166) -> (x-y=w1165:i16)
        "RI relative phase" <- w1165
        n660 = feedback-in #55(w1165) -> ()
        n661 = To Unsigned Byte Integer(number=w1182) -> (unsigned 8bit integer=w1179:u8)
        n662 = feedback #56(u8 0) -> (w1180:u8)
        n663 = Add(x=w1179, y=w1180) -> (x+y=w1178:u8)
        "RI late counter" <- w1178
        n664 = feedback-in #56(w1178) -> ()
        n665 = feedback #57(TRUE) -> (w1159:bool)
        n666 = case shown="2" "Red operating mode" {
          tunnel: [TRUE FALSE w1189] -> w1185
          tunnel: w1159 -> [_ _ w1191]
          frame 0, Default {
          }
          frame 1 {
          }
          frame 2 {
            n667 = Not(x=w1191) -> (.not. x?=w1190:bool)
            n668 = Select(t=w1190, s="Invert RI", f=w1191) -> (s? t:f=w1189:bool)
          }
        }
        n669 = Not(x=w1159) -> (.not. x?=w1160:bool)
        n670 = Select(t="RI ON count", s=w1160, f="RI OFF count") -> (s? t:f=w1171:u16)
        n671 = Subtract(x=w1171, y=w1170) -> (x-y=w1164:u16)
        n672 = Add(x=w1164, y=w1166) -> (x+y=w1158:u16)
        n673 = feedback-in #57(w1160) -> ()
      }
    }
  }
